vi "Multi_Run_Prog.vi"(0 "Command filename":path, 1 "Mode":T9(ring), 2 "Table":T6[](array[typedef]) {"Carrier_2 Q (l/min)" format="%#.2f"; "Row Duration (mins)" format="%#.1f"; "Row No" min=0; "Trace Gas Concentration (%)" min=0.0 format="%#_4f"; "Carrier_1 Q (l/min)" format="%#.2f"; "Tunnel Speed" format="%#.2f"; "Start X" format="%#.2f"; "Start Y" format="%#.2f"; "Start Z" format="%#.2f"; "End X" format="%#.2f"; "End Y" format="%#.2f"; "End Z" format="%#.2f"; "Averaging time (min)" min=0.0 format="%#.2f"}, 3 "Work in Tunnel Coordinates?":T1, 4 "Jump Bad Positions":bool) -> ()   [LabVIEW 2015]
uses:
  Anemometry Sub Vis/Gen Trav/Traverse_cluster.ctl
  Anemometry Sub Vis/Gen Trav/Spacing.ctl
  Anemometry Sub Vis/Controls/Multi_run_mode.ctl
  Anemometry Sub Vis/Gen Trav/Route mapping/Route_Display_Mode.ctl
  Anemometry Sub Vis/Controls/User_Specific_mode.ctl
  Anemometry Sub Vis/Controls/Multi_Run_Case.ctl
  Anemometry Sub Vis/Gen Trav/Multi_Run_Status.ctl
  Anemometry Sub Vis/Controls/Tunnel_Coordinates.ctl
  Anemometry Sub Vis/Controls/Post_Process.ctl
  ADAM Client/Sub VIs/ADAM Controls/Traverse_Level_State.ctl
  ADAM Client/Sub VIs/ADAM Controls/Tunnel_speed_mode.ctl
  Anemometry Sub Vis/Controls/Overhead.ctl
  ADAM Client/Sub VIs/ADAM Controls/Remember_value_mode.ctl
  Anemometry Sub Vis/Gen Trav/Trav_mode.ctl
  Anemometry Sub Vis/Controls/Home.ctl
  ADAM Client/Sub VIs/ADAM Controls/Client_Source_Status.ctl
  ADAM Client/Sub VIs/ADAM Controls/Update_scan_value.ctl
  Anemometry Sub Vis/File/Setup_Filetype.ctl
  Anemometry Sub Vis/Globals/Meas_global.vi
  Anemometry Sub Vis/Globals/Trav_pos_global.vi
  Anemometry Sub Vis/Globals/Preference_global.vi
  Anemometry Sub Vis/Gen Trav/Route mapping/Route_mapping_global.vi
  ADAM Serial/Instrument drivers/Traverses/~subVIs/DriveConfigGlobal.vi
  Anemometry Sub Vis/Globals/Extra_Commands_Global.vi
panel:
  in  "Sort Single\nMeasurements":bool
  out "Last Row Run":i32
  in  "Stop after Repeats":bool
  out "Current Overhead Factor":dbl format="%.3f"
  out "Estimated Completion time":string
  out "Max Tunnel Speed":dbl format="%.2f"
  out "Pause message":string
  in  "Pause":bool
  out "Non Starter":bool
  out "No of Rows":i32
  out "Status":T2
  in  "Synchronization Start No":i32=1 min=1 max=100
  out "Multi Run Case":T3
  out "Simulate/Run":T4
  in  "Display Mode":T5=enum."Display View on Crash"
  in  "stop":bool
  out "Currently on Row":i32
  # "X           Y            Z"
  # "Start"
  # "End"
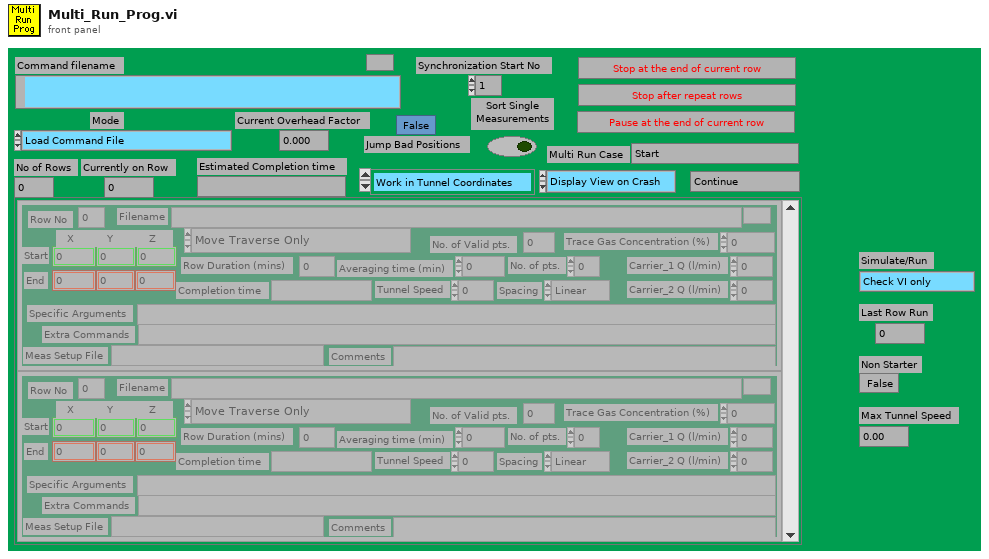
[diagram p1: front panel]
types:
  T1 = typedef "Tunnel_Coordinates.ctl" = enum16{"Work in Tunnel Coordinates", "Work in Model Coordinates"}
  T2 = typedef "Multi_Run_Status.ctl" = enum16{"Continue", "Jump to Next Point", "Jump to Next Row", "Jump To Fall Back", "Terminate Run"}
  T3 = typedef "Multi_Run_Case.ctl" = enum16{"Start", "Load Setup From File", "Has file been edited in Excel?", "Check Max Tunnel Speed", "Pre Check Row", "Check Rows", "Remove blank end rows", "Do results files already exist?", "FFID Bkgnd Measurements?", "First Save Setup file", "Setup Route checking", "Initialise Measurement Prog", "Input Current Position", "Experimental setup control", "Check source flowrates", "Setup for running mode", "Skip Blank Rows", "Which row to execute next", "Evaluate IF Statement", "Perform Measurement Setup", "Set Measurement Conditions", "Execute Row", "Calculate Row TIme", "Update time estimate", "Pause Multi Run Program", "Do Another Row?", "Find Next Fall Back Row", "Shut down source etc", "Email results to users", "Save run efficiency", "Remove Skipped Commands", "Show jumped positions", "Save Setup to File", "End"}
  T4 = typedef "User_Specific_mode.ctl" = enum16{"Check VI only", "Run VI"}
  T5 = typedef "Route_Display_Mode.ctl" = enum16{"Display View Always", "Display View on Crash"}
  T6 = typedef "Traverse_cluster.ctl" = cluster{"Start X":sgl, "Start Y":sgl, "Start Z":sgl, "End X":sgl, "End Y":sgl, "End Z":sgl, "No. of pts.":i32, "Spacing":T7, "Filename":path, "Tunnel Speed":dbl, "Averaging time (min)":dbl, "Extra Commands":string, "Carrier_1 Q (l/min)":dbl, "Carrier_2 Q (l/min)":dbl, "Trace Gas Concentration (%)":dbl, "Specific Arguments":string, "Comments":string, "Row No":i32, "Row Type Selector":T8, "Completion time":string, "Row Duration (mins)":dbl, "No. of Valid pts.":i32, "Meas Setup File":string}
  T7 = typedef "Spacing.ctl" = enum16{"Linear", "Log", "Gauss", "Specified", "N/A"}
  T8 = typedef "Multi_run_mode.ctl" = enum16{"Move Traverse Only", "Set Tunnel Speed Only", "Set Source Only", "Set Measurement Conditions", "Single Measurement", "Vertical Profile", "Lateral Profile", "Longitudinal Profile", "Explore Volume", "Multi-Axis Profile", "Auto Calibrate", "Meas Fast FID Bkgnd", "Check Beam Power", "Scanning Valve Measurement", "Run VI Named:", "Set ADAM Ch", "Wait (minutes)", "Send Message", "Synchronize With:", "Fall Back to this Row", "Turn Off Row Repeating", "Blank Row", "Traverse 3D Volume"}
  T9 = enum16{"Load Command File", "Save Command File", "Check Multi Run Prog", "Check Multi Run Prog With Live Moves", "Run Multi Run Prog"}
  T10 = typedef "Post_Process.ctl" = enum16{"Take New Data", "Post Process Raw Data File"}
  T11 = typedef "Traverse_Level_State.ctl" = enum16{"Running", "Complete"}
  T12 = enum32{"existing file", "new file", "new or existing file", "existing dir", "new dir", "new or existing dir", "existing file (use LLBs)", "new file (use LLBs)", "new or existing file (use LLBs)", "new or existing file or directory (use LLBs)"}
  T13 = typedef "Tunnel_speed_mode.ctl" = enum16{"Set Speed", "Set Speed then wait", "Is tunnel speed allowable?"}
  T14 = enum16{"All Channel Names", "Valid Channel Names"}
  T15 = typedef "Overhead.ctl" = enum16{"Update total times", "Read Current Overhead", "Re Scale totals to 3 hrs", "Initialise totals to 3hr"}
  T16 = typedef "Remember_value_mode.ctl" = enum16{"Read only", "Read and Write"}
  T17 = typedef "Home.ctl" = enum16{"Don't Home", "Home  +X", "Home  -X", "Home  +Y", "Home  -Y", "Home  +Z", "Home  -Z"}
  T18 = typedef "Trav_mode.ctl" = enum16{"Move traverse", "Read traverse position", "Teach Position"}
  T19 = typedef "Client_Source_Status.ctl" = enum16{"Not Using", "Using", "Must Have"}
  T20 = typedef "Update_scan_value.ctl" = cluster{"Channel Name":string, "New Value":dbl}
  T21 = typedef "Setup_Filetype.ctl" = enum16{"Measurement Setups", "Calibration Setups", "General", "Results File Plotter Setups", "Speed Calib Tweaks"}
  T22 = typedef "AxisConfigCluster.ctl" = cluster{"Channel Properties":T23, "Static Drive Configuration":T24}
  T23 = typedef "DriveProperties.ctl" = cluster{"Channel Name":string, "Vel. Default":sgl, "Acc. Default":sgl, "Vel. Max":sgl, "Vel. Min":sgl, "Acc. Max":sgl, "Acc. Min":sgl, "Pulses/unit":sgl, "Address":u8, "Pulse Offset":i32, "Pos Tolerance":sgl, "Pulses/rev":sgl, "Backlash/Eng units":sgl, "Current Pos":sgl, "Ch Status":enum16{"Active", "Offline", "Simulate"}, "Port Name":string, "Axis Transform mode":string, "Metadata Ch Name":string, "Type":string}
  T24 = typedef "DriveStaticConfig.ctl" = cluster{"Correction Gain % (CG)":u16, "Dead Band (DB)":i32, "Dead Band Window (DW)":i32, "Encoder Resolution (ER)":i32, "Step Mode  (FSB)":u16, "Position Maintenance (FSC)":u16, "Stop on Stall (FSD)":u16, "Activate OP1 on stall (FSE)":u16, "Stop on Trigger 3 (FSF)":u16, "OP2 in Deadband (FSG)":u16, "Stall Detect (FSH)":u16, "Limit Disable (LD)":u16, "Motor Resolution (MR)":enum16{"200", "400", "1000", "2000", "4000", "5000", "10000", "12800", "18000", "20000", "21600", "25000", "25400", "25600", "36000", "50000", "278528", "425984", "507904", "614400", "655360", "819200", "1024000"}, "Limit Switch Sense (OSA)":u16, "Home Position (OSB)":u16, "Home Switch Sense (OSC)":u16, "Encoder Z for Home (OSD)":u16, "Reference edge of Home (OSH)":u16, "RS232 Echo Control (SSA)":u16, "Buffer at Limit (SSG)":u16, "Buffer at Stop (SSH)":u16, "Indexer Mode  (FSA)":u16, "Type":string, "ConfigString":string, "De Power Motor":enum16{"TRUE", "FALSE"}}
  T25 = typedef "Status_Cluster.ctl" = cluster{"Status":T2, "Error Type":string, "Error Description":string}
  T26 = typedef "Server_Comms.ctl" = enum16{"Server Link Healthy", "Do Not Link To Server"}
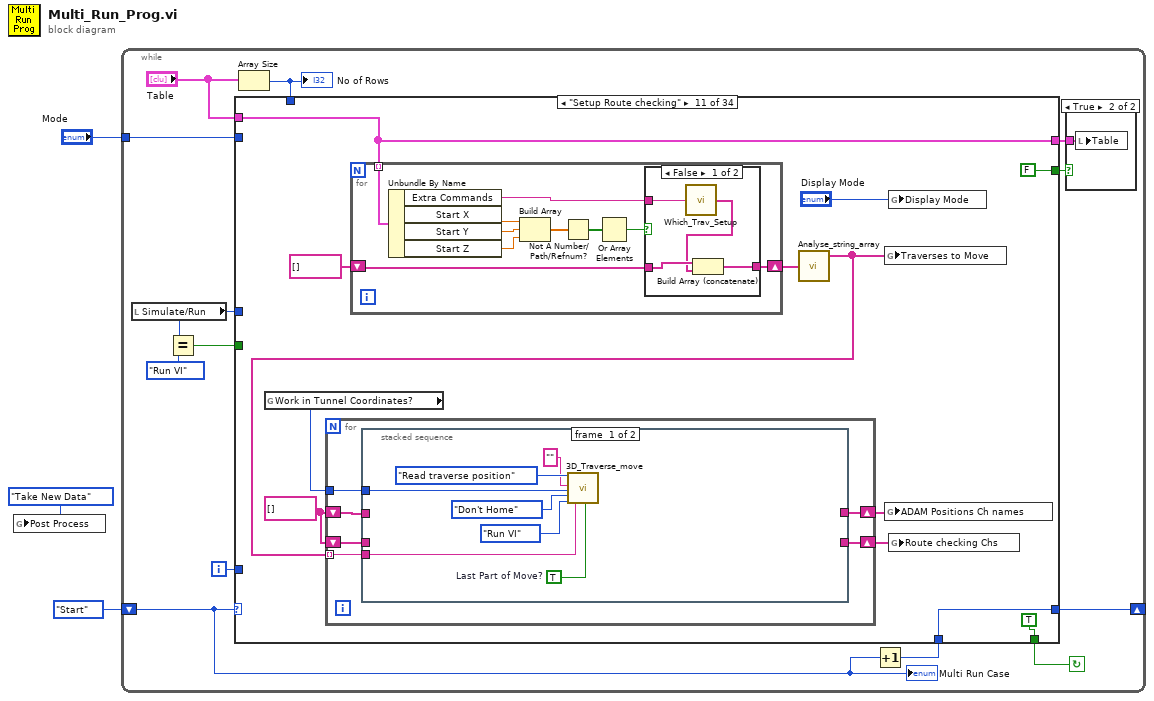
[diagram p0: block diagram]
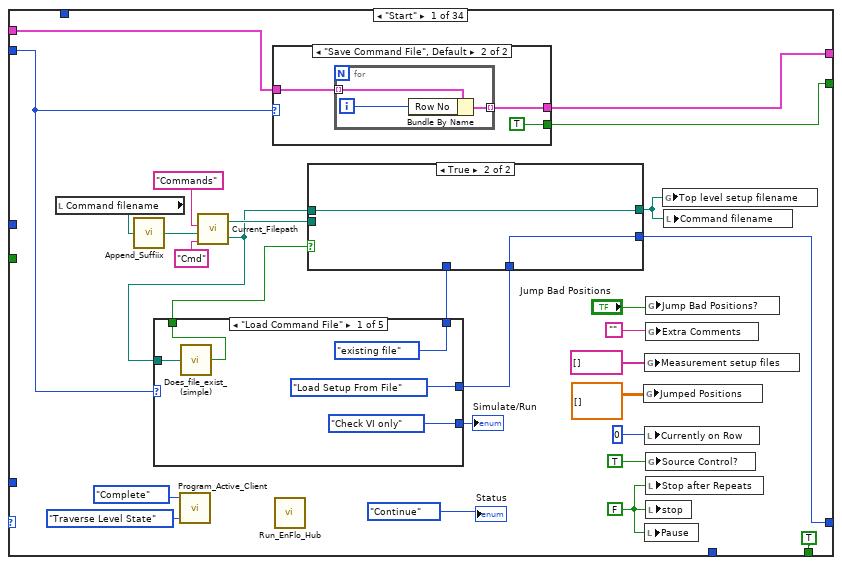
[diagram p3: hidden frame]
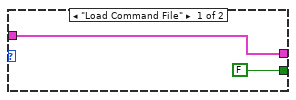
[diagram p4: hidden frame]
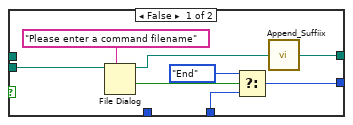
[diagram p5: hidden frame]
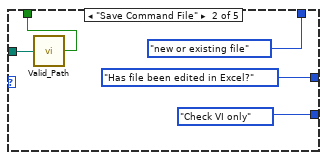
[diagram p6: hidden frame]
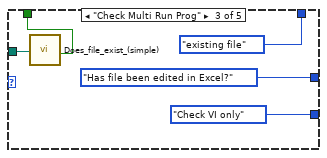
[diagram p7: hidden frame]
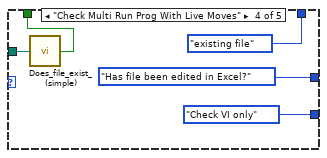
[diagram p8: hidden frame]
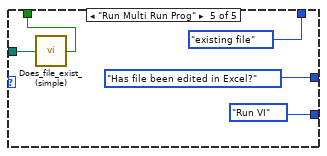
[diagram p9: hidden frame]
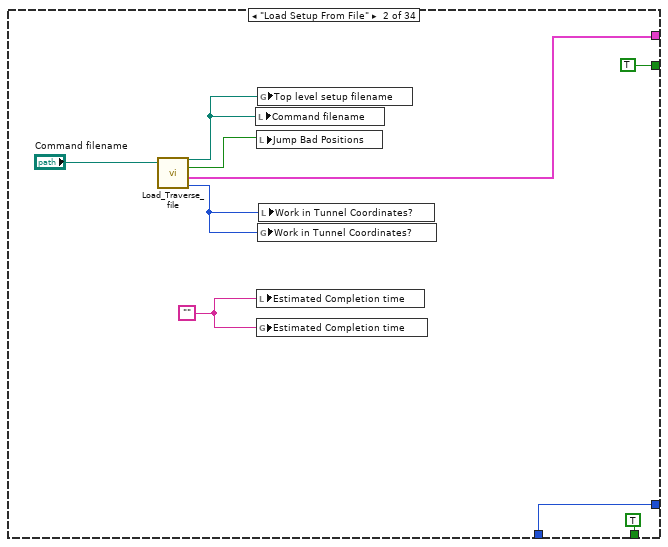
[diagram p10: hidden frame]
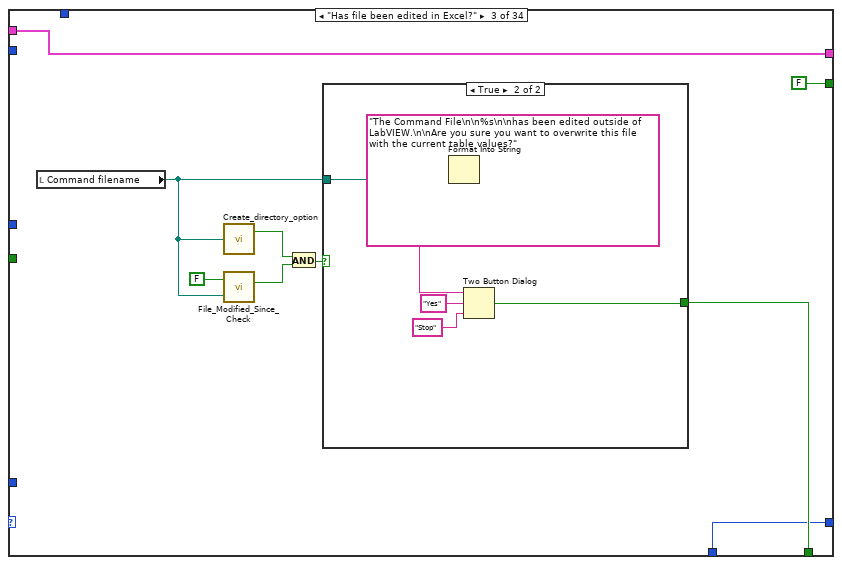
[diagram p11: hidden frame]
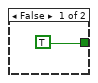
[diagram p12: hidden frame]
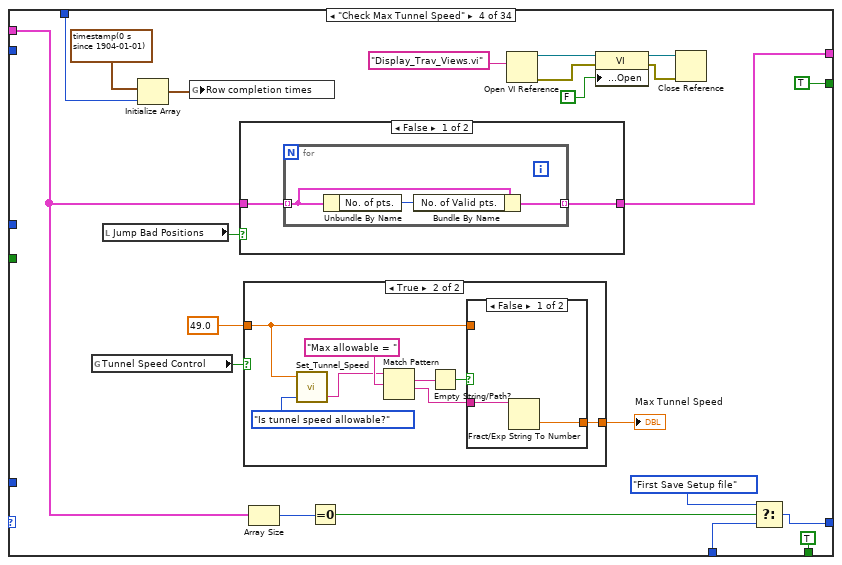
[diagram p13: hidden frame]
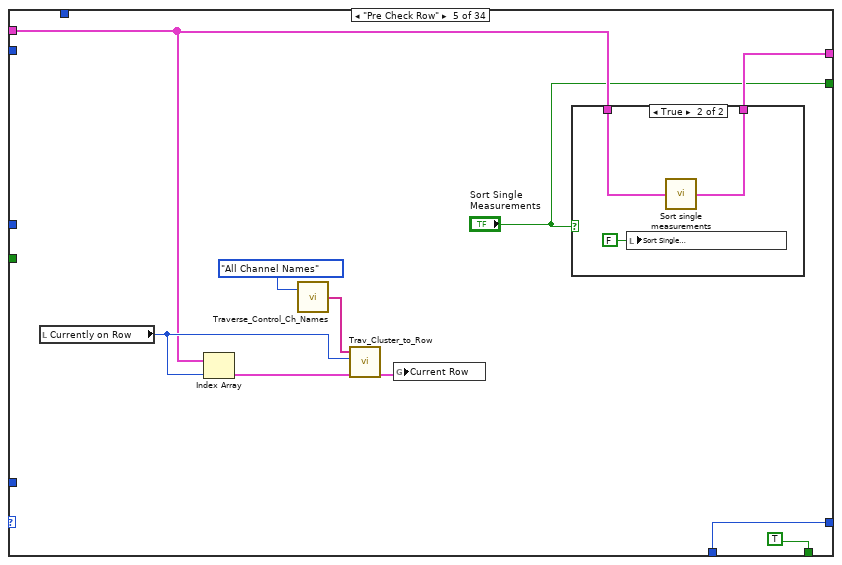
[diagram p17: hidden frame]
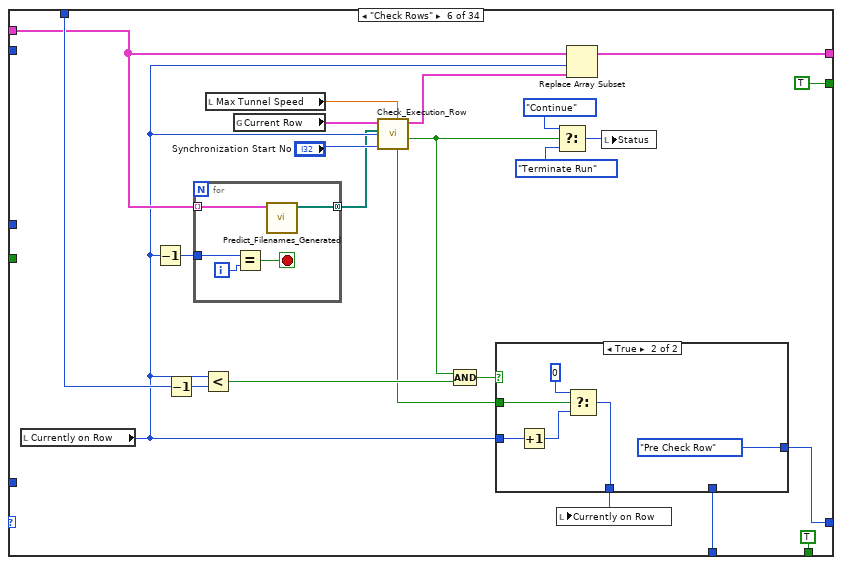
[diagram p19: hidden frame]
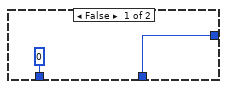
[diagram p20: hidden frame]
diagram:
  n1 = global write "Meas_global.vi" "Post Process"(Post_Process."Take New Data" ("Post Process")) -> ()
  n2 = while {
    shift-left: Multi_Run_Case."Start" ("Multi Run Case") -> [w12]
    shift-right: [w9] -> _
    tunnel: "Mode" -> [w15]
    i -> [w13]
    stop <- w16 continue-if-true
    n3 = local read "Simulate/Run"() -> (w5:T4)
    n4 = Equal?(x=w5, y=User_Specific_mode."Run VI" ("Simulate/Run")) -> (x = y?=w4:bool)
    n5 = Array Size(array="Table") -> (size(s)=w8:i32)
    "No of Rows" <- w8
    n6 = Increment(x=w12) -> (x+1=w14:T3)
    n7 = case shown="\"Setup Route checking\"" w12 {
      tunnel: [TRUE TRUE w100 TRUE TRUE TRUE TRUE TRUE TRUE TRUE TRUE ("Continue?") TRUE ("Continue?") TRUE TRUE TRUE w545 TRUE ("Continue?") TRUE ("Continue?") TRUE TRUE ("Continue?") TRUE TRUE TRUE TRUE TRUE TRUE TRUE TRUE TRUE TRUE TRUE TRUE TRUE FALSE] -> w16
      tunnel: w15 -> [w30 _ _ _ _ _ _ _ _ w426 _ _ _ _ _ _ _ _ _ _ _ _ _ _ _ _ _ _ _ _ _ _ w1268 _]
      tunnel: "Table" -> [w42 _ w97 w127 w155 w170 w204 w235 w393 w428 w451 w507 w519 w526 w534 w548 w610 w654 w758 w809 w821 w911 w945 w977 w1020 w1064 w1109 w1138 w1163 w1210 w1215 w1224 w1287 w1350]
      tunnel: w5 -> [_ _ _ _ _ _ _ w234 _ _ _ _ _ _ w533 w547 _ w652 _ w806 w818 w910 _ w974 _ w1070 _ _ _ _ _ _ w1278 _]
      tunnel: w14 -> [_ w93 w99 w125 w161 w176 w215 w238 w390 w425 w454 w505 w520 w525 w538 w550 w612 w650 w763 w810 w828 w908 w938 w979 w1023 _ _ w1124 w1165 w1212 w1218 w1232 w1285 w1349]
      tunnel: w13 -> [_ _ _ _ _ _ _ _ _ _ _ _ _ _ _ _ _ _ _ _ _ _ _ _ w1021 _ _ _ _ _ _ _ _ _]
      tunnel: [w40 w93 w99 w124 w161 w175 w215 w238 w390 w421 w454 w504 w520 w525 w536 w550 w612 w651 w762 w810 w829 w908 w938 w979 w1024 w1059 w1107 w1133 w1165 w1212 w1218 w1232 w1285 w1349] -> w9
      tunnel: [w29 TRUE FALSE ("Rows Added ?") TRUE ("Rows Added ?") "Sort Single\nMeasurements" TRUE TRUE FALSE FALSE TRUE FALSE FALSE FALSE FALSE FALSE TRUE FALSE ("Rows Added ?") FALSE ("Rows Added ?") FALSE FALSE ("Rows Added ?") FALSE FALSE FALSE TRUE ("Rows Added ?") FALSE FALSE FALSE FALSE FALSE FALSE TRUE TRUE TRUE FALSE] -> w10
      tunnel: w8 -> [_ _ _ w119 _ w180 w206 _ _ _ _ _ _ _ _ _ w613 w653 _ _ _ _ _ w973 _ w1062 w1100 _ _ _ _ _ w1259 _]
      tunnel: [w41 w94 w97 w129 w154 w183 w210 w235 w393 w429 w451 w507 w519 w526 w534 w546 w610 w655 w758 w809 w821 w911 w945 w976 w1020 w1064 w1109 w1138 w1163 w1210 w1214 w1224 w1286 w1350] -> w7
      tunnel: w4 -> [_ _ _ _ _ _ _ _ _ _ _ _ _ w523 w532 _ _ _ w752 _ _ _ w937 _ _ _ _ _ _ _ _ _ _ _]
      frame "Start" {
        w27 = FALSE ("Measurment setup Found?")
        n8 = local read "Command filename"() -> (w32:path)
        n9 = call "Append_Suffiix.vi"("Results file"=w32) -> ("appended path"=w22:path)
        n10 = call "Program_Active_Client.vi"("Mode"=enum16{"Program Active", "Traverse Level State"}."Traverse Level State", "Traverse level State"=Traverse_Level_State."Complete") -> ()  [unwired: 1 in, 3 out]
        n11 = call "Current_Filepath.vi"("Short_Name"="Cmd" ("Data Type"), "Filename in"=w22, "Data Type"="Commands") -> ("Filename Out"=w19:path, "Directory"=w21:path)  [unwired: 1 in]
        n12 = case shown="\"Load Command File\"" w30 {
          tunnel: [User_Specific_mode."Check VI only" ("Simulate/Run") User_Specific_mode."Check VI only" ("Simulate/Run") User_Specific_mode."Check VI only" ("Simulate/Run") User_Specific_mode."Check VI only" ("Simulate/Run") User_Specific_mode."Run VI" ("Simulate/Run")] -> w43
          tunnel: [Multi_Run_Case."Load Setup From File" ("Multi Run Case") Multi_Run_Case."Has file been edited in Excel?" ("Multi Run Case") Multi_Run_Case."Has file been edited in Excel?" ("Multi Run Case") Multi_Run_Case."Has file been edited in Excel?" ("Multi Run Case") Multi_Run_Case."Has file been edited in Excel?" ("Multi Run Case")] -> w39
          tunnel: [T12."existing file" ("select mode (2)") T12."new or existing file" ("select mode (2)") T12."existing file" ("select mode (2)") T12."existing file" ("select mode (2)") T12."existing file" ("select mode (2)")] -> w28
          tunnel: w19 -> [w64 w69 w73 w79 w84]
          tunnel: [w63 w68 w74 w78 w83] -> w18
          frame "Load Command File" {
            n13 = call "Does_file_exist_(simple).vi"("Pathname"=w64) -> ("exists?"=w63:bool)
          }
          frame "Save Command File" {
            n14 = call "Valid_Path.vi"("Filename"=w69) -> ("Valid Path?"=w68:bool)
          }
          frame "Check Multi Run Prog" {
            n15 = call "Does_file_exist_(simple).vi"("Pathname"=w73) -> ("exists?"=w74:bool)
          }
          frame "Check Multi Run Prog With Live Moves" {
            n16 = call "Does_file_exist_(simple).vi"("Pathname"=w79) -> ("exists?"=w78:bool)
          }
          frame "Run Multi Run Prog" {
            n17 = call "Does_file_exist_(simple).vi"("Pathname"=w84) -> ("exists?"=w83:bool)
          }
        }
        "Simulate/Run" <- w43
        n18 = case shown="\"Save Command File\", Default" w30 {
          tunnel: w42 -> [w46 w49]
          tunnel: [w46 w48] -> w41
          tunnel: [FALSE TRUE] -> w29
          frame "Load Command File" {
          }
          frame "Save Command File", Default {
            n19 = for {
              tunnel: w49 -> [w52] mode=indexing
              tunnel: [w51] -> w48 mode=indexing
              i -> [w50]
              n20 = Bundle By Name(cluster=w52, "Row No"=w50) -> (w51:T6)
            }
          }
        }
        n21 = call "Run_EnFlo_Hub.vi"() -> ()  [unwired: 8 out]
        n22 = case shown="True" w18 {
          tunnel: [w58 w62] -> w40
          tunnel: w39 -> [w59 w62]
          tunnel: w19 -> [_ w61]
          tunnel: [w57 w61] -> w31
          tunnel: w28 -> [_ _]
          tunnel: w21 -> [w53 _]
          frame False {
            n23 = File Dialog(7:"Please enter a command filename" ("prompt"), 11:w53) -> (1:w55:bool, 3:w56:path)  [unwired: 1 in, 6 out]
            n24 = Select(t=Multi_Run_Case."End" ("Multi Run Case"), s=w55, f=w59) -> (s? t:f=w58:T3)
            n25 = call "Append_Suffiix.vi"("Results file"=w56) -> ("appended path"=w57:path)
          }
          frame True {
          }
        }
        n26 = global write "Trav_pos_global.vi" "Jumped Positions"(dbl[][] [] ("Jumped Positions")) -> ()
        n27 = global write "Trav_pos_global.vi" "Measurement setup files"(string[] [] ("Measurement setup files")) -> ()
        n28 = local write "Currently on Row"(0 ("Currently on Row")) -> ()
        n29 = local write "Pause"(w27) -> ()
        n30 = global write "Trav_pos_global.vi" "Jump Bad Positions?"("Jump Bad Positions") -> ()
        n31 = global write "Meas_global.vi" "Extra Comments"("") -> ()
        n32 = global write "Trav_pos_global.vi" "Source Control?"(TRUE ("Source Control?")) -> ()
        n33 = local write "Stop after Repeats"(w27) -> ()
        n34 = local write "stop"(w27) -> ()
        n35 = global write "Trav_pos_global.vi" "Top level setup filename"(w31) -> ()
        n36 = local write "Command filename"(w31) -> ()
        "Status" <- Multi_Run_Status."Continue" ("Status")
      }
      frame "Load Setup From File" {
        w89 = ""
        n37 = call "Load_Traverse_file.vi"("Setup filename"="Command filename") -> ("Setup filename Out"=w91:path, "Jump Bad Positions"=w88:bool, "Table"=w94:T6[], "Work in Tunnel Coordinates?"=w90:T1)  [unwired: 2 out]
        n38 = local write "Command filename"(w91) -> ()
        n39 = local write "Jump Bad Positions"(w88) -> ()
        n40 = local write "Estimated Completion time"(w89) -> ()
        n41 = global write "Trav_pos_global.vi" "Estimated Completion time"(w89) -> ()
        n42 = global write "Trav_pos_global.vi" "Top level setup filename"(w91) -> ()
        n43 = global write "Trav_pos_global.vi" "Work in Tunnel Coordinates?"(w90) -> ()
        n44 = local write "Work in Tunnel Coordinates?"(w90) -> ()
      }
      frame "Has file been edited in Excel?" {
        n45 = local read "Command filename"() -> (w101:path)
        n46 = call "Create_directory_option.vi"("Filename"=w101) -> ("Path is to existing File"=w104:bool)  [unwired: 1 out]
        n47 = call "File_Modified_Since_Check.vi"("Pathname"=w101, "Just Modified?"=FALSE) -> ("Modified?"=w103:bool)
        n48 = And(x=w104, y=w103) -> (x .and. y?=w105:bool)
        n49 = case shown="True" w105 {
          tunnel: w101 -> [_ w112]
          tunnel: [TRUE ("T button?") w107] -> w100
          frame False {
          }
          frame True {
            n50 = Format Into String(format string="The Command File\n\n%s\n\nhas been edited outside of LabVIEW.\n\nAre you sure you want to overwrite this file  with the current table values?" ("Format String"), w112) -> (resulting string=w110:string)  [unwired: 2 in, 1 out]
            n51 = Two Button Dialog(message=w110, 1:"Stop" ("F button name (\"Cancel\")"), 2:"Yes" ("T button name (\"OK\")")) -> (T button?=w107:bool)
          }
        }
      }
      frame "Check Max Tunnel Speed" {
        n52 = global read "Preference_global.vi" "Tunnel Speed Control"() -> (w130:bool)
        n53 = local read "Jump Bad Positions"() -> (w128:bool)
        n54 = Initialize Array(timestamp(0 s since 1904-01-01) ("seconds since 1Jan1904"), w119) -> (w120:timestamp[])
        n55 = global write "Trav_pos_global.vi" "Row completion times"(w120) -> ()
        n56 = case shown="False" w128 {
          tunnel: w127 -> [w136 w140]
          tunnel: [w135 w140] -> w129
          frame False {
            n57 = for {
              tunnel: w136 -> [w138] mode=indexing
              tunnel: [w137] -> w135 mode=indexing
              n58 = Unbundle By Name(w138) -> ("No. of pts."=w139:i32)
              n59 = Bundle By Name(cluster=w138, "No. of Valid pts."=w139) -> (w137:T6)
            }
          }
          frame True {
          }
        }
        n60 = case shown="True" w130 {
          tunnel: 49.0 ("Tunnel Velocity m/s") -> [w141 w142]
          tunnel: [w141 w144] -> w132
          frame False {
          }
          frame True {
            n61 = call "Set_Tunnel_Speed.vi"("Mode"=Tunnel_speed_mode."Is tunnel speed allowable?", "Tunnel Velocity m/s"=w142) -> ("Error String"=w147:string)  [unwired: 1 in, 2 out]
            n62 = Match Pattern(string=w147, regular expression="Max allowable = ") -> (match substring=w146:string, after substring=w143:string)  [unwired: 3 out]
            n63 = Empty String/Path?(string/path=w146) -> (empty?=w145:bool)
            n64 = case shown="False" w145 {
              tunnel: [w150 w152] -> w144
              tunnel: w142 -> [_ w152]
              tunnel: w143 -> [w151 _]
              frame False {
                n65 = Fract/Exp String To Number(string=w151) -> (number=w150:dbl)  [unwired: 4 out]
              }
              frame True {
              }
            }
          }
        }
        "Max Tunnel Speed" <- w132
        n66 = Array Size(array=w127) -> (size(s)=w126:i32)
        n67 = Equal To 0?(x=w126) -> (x = 0?=w123:bool)
        n68 = Open VI Reference(vi path="Display_Trav_Views.vi" ("VI path")) -> (vi reference=w118:refnum<vi>, error out=w117:errorcluster)  [unwired: 1 in, 4 out]
        n69 = property class="VI"(reference=w118, error in=w117, "Front Panel Window:Open"=FALSE) -> (reference out=w115:refnum<vi>, error out=w114:errorcluster)
        n70 = Close Reference(reference=w115, error in (no error)=w114) -> ()  [unwired: 1 out]
        n71 = Select(t=Multi_Run_Case."First Save Setup file" ("Multi Run Case"), s=w123, f=w125) -> (s? t:f=w124:T3)
      }
      frame "Pre Check Row" {
        n72 = local read "Currently on Row"() -> (w158:i32)
        n73 = Index Array(array=w155, index=w158) -> (element=w159:T6)
        n74 = call "Traverse_Control_Ch_Names.vi"("Mode"=T14."All Channel Names") -> ("Channel names"=w156:string[])  [unwired: 1 in]
        n75 = call "Trav_Cluster_to_Row.vi"("Traverse line in"=w159, "Row Number"=w158, "Channel names"=w156) -> ("Traverse line Out"=w160:T6)  [unwired: 4 out]
        n76 = global write "Trav_pos_global.vi" "Current Row"(w160) -> ()
        n77 = case shown="True" "Sort Single\nMeasurements" {
          tunnel: w155 -> [w163 w166]
          tunnel: [w163 w165] -> w154
          frame False {
          }
          frame True {
            n78 = local write "Sort Single\nMeasurements"(FALSE ("Sort Single\nMeasurements")) -> ()
            n79 = call "Sort single measurements.vi"("Table In"=w166) -> ("Table Out"=w165:T6[])
          }
        }
      }
      frame "Check Rows" {
        n80 = local read "Currently on Row"() -> (w169:i32)
        n81 = Decrement(x=w169) -> (x-1=w168:i32)
        n82 = Decrement(x=w180) -> (x-1=w173:i32)
        n83 = for {
          tunnel: w170 -> [w194] mode=indexing
          tunnel: w168 -> [w192]
          tunnel: [w190] -> w167 mode=concatenating
          i -> [w193]
          stop <- w191 stop-if-true
          n84 = Equal?(x=w192, y=w193) -> (x = y?=w191:bool)
          n85 = call "Predict_Filenames_Generated.vi"("Traverse line"=w194) -> ("Filename"=w190:path[])  [unwired: 10 in]
        }
        n86 = Less?(x=w169, y=w173) -> (x < y?=w179:bool)
        n87 = local read "Max Tunnel Speed"() -> (w182:dbl)
        n88 = global read "Trav_pos_global.vi" "Current Row"() -> (w171:T6)
        n89 = call "Check_Execution_Row.vi"("Execution Row"=w171, "Earlier Filenames"=w167, "Synchronization Start No"="Synchronization Start No", "Row Index"=w169, "Max Tunnel Speed"=w182) -> ("Edited Row"=w172:bool, "Execution Row Out"=w174:T6, "Continue?"=w181:bool)  [unwired: 3 out]
        n90 = Compound Arithmetic op=AND(w181, w179) -> (w178:bool)
        n91 = case shown="True" w178 {
          tunnel: [0 w198] -> w177
          tunnel: w169 -> [_ w202]
          tunnel: w176 -> [w196 _]
          tunnel: [w196 Multi_Run_Case."Pre Check Row" ("Multi Run Case")] -> w175
          tunnel: w172 -> [_ w200]
          frame False {
          }
          frame True {
            n92 = Increment(x=w202) -> (x+1=w199:i32)
            n93 = Select(t=0, s=w200, f=w199) -> (s? t:f=w198:i32)
          }
        }
        n94 = Select(t=Multi_Run_Status."Continue" ("Status"), s=w181, f=Multi_Run_Status."Terminate Run" ("Status")) -> (s? t:f=w187:T2)
        n95 = local write "Currently on Row"(w177) -> ()
        n96 = Replace Array Subset(array=w170, new element=w174, index=w169) -> (w183:T6[])
        n97 = local write "Status"(w187) -> ()
      }
      frame "Remove blank end rows" {
        n98 = local read "Jump Bad Positions"() -> (w203:bool)
        n99 = case shown="False" w203 {
          tunnel: w206 -> [w221 _]
          tunnel: w204 -> [w220 w224]
          tunnel: [w218 w224] -> w205
          frame False {
            n100 = call "Calc_Remaining_Time.vi"("Currently on Row"=-1 ("Start Index"), "Table In"=w220) -> ("Table Out"=w218:T6[])  [unwired: 1 out]
            n101 = Decrement(x=w221) -> (x-1=w223:i32)
            n102 = Index Array(array=w218, index=w223) -> (element=w222:T6)
            n103 = Unbundle By Name(w222) -> ("Completion time"=w217:string)
            n104 = global write "Trav_pos_global.vi" "Estimated Completion time"(w217) -> ()
            n105 = local write "Estimated Completion time"(w217) -> ()
          }
          frame True {
          }
        }
        n106 = Reverse 1D Array(array=w205) -> (reversed array=w214:T6[])
        n107 = while {
          tunnel: [w225] -> w212
          tunnel: w206 -> [w229]
          tunnel: w214 -> [w233] mode=indexing
          i -> [w225]
          stop <- w226 continue-if-true
          n108 = Unbundle By Name(w233) -> ("Row Type Selector"=w231:T8)
          n109 = Increment(x=w225) -> (x+1=w230:i32)
          n110 = Greater?(x=w229, y=w230) -> (0:w228:bool)
          n111 = Equal?(x=Multi_run_mode."Blank Row" ("Row Type Selector"), y=w231) -> (x = y?=w227:bool)
          n112 = And(x=w227, y=w228) -> (x .and. y?=w226:bool)
        }
        n113 = Subtract(x=w206, y=w212) -> (x-y=w211:i32)
        n114 = call "Overhead_Factor.vi"("Mode"=Overhead."Read Current Overhead") -> ("Current Overhead Factor"=w207:dbl)  [unwired: 3 in]
        n115 = local write "Current Overhead Factor"(w207) -> ()
        n116 = Array Subset(array=w205, index=0 ("Array Index"), length=w211) -> (w210:T6[])
      }
      frame "Do results files already exist?" {
        n117 = for {
          tunnel: w235 -> [w247] mode=indexing
          shift-right: [w243] -> _
          shift-left: path[] [] -> [w244]
          tunnel: w234 -> [w241]
          n118 = Unbundle By Name(w247) -> ("Specific Arguments"=w240:string, "Row Type Selector"=w246:T8, "Filename"=w245:path)
          n119 = while {
            shift-left: w244 -> [w255]
            shift-right: [w254] -> w243
            tunnel: w245 -> [w256]
            tunnel: w246 -> [w260]
            shift-left: 0 -> [w261]
            shift-right: [w257] -> _
            tunnel: w241 -> [w251]
            shift-right: [w250] -> _
            shift-left: _ -> [w249]
            tunnel: w240 -> [w248]
            stop <- w259 continue-if-true
            n120 = Increment(x=w261) -> (x+1=w258:i32)
            n121 = case shown="0, Default" w261 {
              tunnel: w260 -> [w270 _ _ _ _ _ _ _ _ _ _ _]
              tunnel: [w265 w292 w297 w304 w309 TRUE ("exists?") TRUE ("exists?") FALSE ("exists?") FALSE ("exists?") TRUE ("true") w366 w379] -> w259
              tunnel: w258 -> [w272 w295 w300 w303 w310 w315 w326 w337 w348 w352 w364 _]
              tunnel: [w272 w295 w300 w303 w310 w313 w325 w337 w348 w353 w364 w378] -> w257
              tunnel: [w271 w294 w299 w302 w307 w323 w334 w339 w341 w350 w368 w384] -> w254
              tunnel: w255 -> [w271 w294 w299 w302 w308 w323 w334 w339 w341 w350 w368 w384]
              tunnel: w256 -> [w264 _ _ _ _ _ _ _ _ _ _ _]
              tunnel: 7 -> [_ _ _ _ _ _ _ _ _ w351 _ w378]
              tunnel: 9 -> [_ _ _ _ _ w314 _ _ _ _ _ _]
              tunnel: w251 -> [_ _ _ _ _ _ _ _ _ _ w367 _]
              tunnel: [w263 w291 w296 w301 w306 w311 w324 w335 w340 w349 w365 w377] -> w250
              tunnel: w249 -> [_ w291 w296 w301 w306 w311 w324 w335 w340 w349 w365 w377]
              tunnel: w248 -> [w262 _ _ _ _ _ _ _ _ _ _ _]
              frame 0, Default {
                n122 = case shown="\"Run VI Named:\"" w270 {
                  tunnel: [TRUE w283 FALSE FALSE] -> w267
                  tunnel: w264 -> [w273 w282 w287 w289]
                  tunnel: w262 -> [_ w280 _ _]
                  tunnel: [w273 w282 w287 w289] -> w263
                  frame "Move Traverse Only", Default {
                  }
                  frame "Run VI Named:" {
                    n123 = Match Pattern(string=w280, regular expression=";") -> (before substring=w279:string)  [unwired: 4 out]
                    n124 = call <vilib>:"Trim Whitespace.vi"("string"=w279) -> ("trimmed string"=w277:string)  [unwired: 1 in]
                    n125 = Equal?(x=w277, y="Pressure_Tapped_Cube.vi") -> (x = y?=w284:bool)
                    n126 = Equal?(x=w277, y="Take_Data_on_the_Move.vi") -> (x = y?=w278:bool)
                    n127 = Equal?(x=w277, y="Capture_Flow_Vis.vi") -> (x = y?=w275:bool)
                    n128 = Compound Arithmetic op=OR(w284, w278, w275) -> (w283:bool)
                  }
                  frame "Auto Calibrate" {
                  }
                  frame "Send Message" {
                  }
                }
                n129 = local read "Status"() -> (w268:T2)
                n130 = Not Equal?(x=Multi_Run_Status."Terminate Run" ("Status"), y=w268) -> (x != y?=w266:bool)
                n131 = And(x=w267, y=w266) -> (x .and. y?=w265:bool)
              }
              frame 1 {
                n132 = Not Equal?(x=path "", y=w291) -> (x != y?=w292:bool)
              }
              frame 2 {
                n133 = Not Equal?(x=w296, y=path "") -> (x != y?=w297:bool)
              }
              frame 3 {
                n134 = Search 1D Array(1D array=w302, element=w301) -> (index of element=w305:i32)  [unwired: 1 out]
                n135 = Less Than 0?(x=w305) -> (x < 0?=w304:bool)
              }
              frame 4 {
                n136 = Build Array (concatenate)(w308, w306) -> (w307:path[])
                n137 = call "Does_file_exist_(simple).vi"("Pathname"=w306) -> ("exists?"=w309:bool)
              }
              frame 5 {
                n138 = Path To String(path=w311) -> (string=w322:string)
                n139 = global read "Meas_global.vi" "Start Time of experiment"() -> (w317:dbl)
                n140 = Concatenate Strings(w322, "Append" ("Substring")) -> (w320:string)
                n141 = call "Remember_value.vi"("Mode"=Remember_value_mode."Read only", "Ch name"=w320) -> ("Output Value"=w318:dbl)  [unwired: 1 in]
                n142 = Not Equal?(x=w317, y=w318) -> (x != y?=w316:bool)
                n143 = Select(t=w315, s=w316, f=w314) -> (s? t:f=w313:i32)
              }
              frame 6 {
                n144 = Increment(x=w326) -> (x+1=w327:i32)
                n145 = Format Into String(format string="The results filename \"%s\" already exists.\nDo you wish to append to this file during the run?" ("Format String"), w324) -> (resulting string=w331:string)  [unwired: 2 in, 1 out]
                n146 = Two Button Dialog(message=w331, 1:"Abort Run" ("F button name (\"Cancel\")"), 2:"Append" ("T button name (\"OK\")")) -> (T button?=w328:bool)
                n147 = Select(t=w327, s=w328, f=w326) -> (s? t:f=w325:i32)
              }
              frame 7 {
                n148 = local write "Status"(Multi_Run_Status."Terminate Run" ("Status")) -> ()
              }
              frame 8 {
                n149 = Path To String(path=w340) -> (string=w347:string)
                n150 = Concatenate Strings(w347, "Append" ("Substring")) -> (w345:string)
                n151 = global read "Meas_global.vi" "Start Time of experiment"() -> (w342:dbl)
                n152 = call "Remember_value.vi"("Mode"=Remember_value_mode."Read and Write", "Input Value"=w342, "Ch name"=w345) -> ()  [unwired: 1 out]
              }
              frame 9 {
                n153 = call "Read_File_Simple.vi"("Filename"=w349) -> ("string"=w356:string)  [unwired: 2 in, 7 out]
                n154 = call "Is_it_a_Results_File.vi"("character string"=w356) -> ("Results File?"=w355:bool)  [unwired: 2 out]
                n155 = case shown="False" w355 {
                  tunnel: w349 -> [w359 _]
                  tunnel: [w357 w363] -> w353
                  tunnel: w352 -> [_ w363]
                  tunnel: w351 -> [w357 _]
                  frame False {
                    n156 = Path To String(path=w359) -> (string=w361:string)
                    n157 = Format Into String(format string="The File %s is not in the correct Results file format.\nCheck that it is tab delimited rather than excel format, or choose another file." ("Format String"), w361) -> (resulting string=w358:string)  [unwired: 2 in, 1 out]
                    n158 = One Button Dialog(message=w358, button name ("OK")="Stop") -> ()  [unwired: 1 out]
                  }
                  frame True {
                  }
                }
              }
              frame 10 {
                n159 = case shown="\"Run VI\"" w367 {
                  tunnel: w365 -> [_ w376]
                  tunnel: [FALSE ("exists?") w370] -> w366
                  frame "Check VI only", Default {
                  }
                  frame "Run VI" {
                    n160 = call "Open_File_for_write.vi"("append to file? (new file:F)"=TRUE, "file path"=w376) -> ("error out"=w374:errorcluster, "refnum"=w375:refnum<file>)  [unwired: 1 in, 7 out]
                    n161 = Unbundle By Name(w374) -> ("code"=w373:i32)
                    n162 = Close File(refnum=w375, error in=w374) -> ()  [unwired: 2 out]
                    n163 = Equal?(x=10 ("code"), y=w373) -> (x = y?=w370:bool)
                  }
                }
              }
              frame 11 {
                n164 = Path To String(path=w377) -> (string=w382:string)
                n165 = Format Into String(format string="The File %s is already open in another application." ("Format String"), w382) -> (resulting string=w381:string)  [unwired: 2 in, 1 out]
                n166 = One Button Dialog(message=w381, button name ("OK")="Stop") -> (true=w379:bool)
              }
            }
          }
        }
      }
      frame "FFID Bkgnd Measurements?" {
        n167 = for {
          tunnel: w393 -> [w406] mode=indexing
          tunnel: [w404] -> w392 mode=indexing
          tunnel: [w403] -> w391 mode=indexing
          tunnel: [w401] -> w386 mode=indexing
          n168 = Unbundle By Name(w406) -> ("Specific Arguments"=w402:string, "Carrier_1 Q (l/min)"=w399:dbl, "Carrier_2 Q (l/min)"=w398:dbl, "Row Type Selector"=w400:T8)
          n169 = Add(x=w399, y=w398) -> (x+y=w397:dbl)
          n170 = case shown="\"Auto Calibrate\"" w400 {
            tunnel: w397 -> [w409 _]
            tunnel: [FALSE w410] -> w403
            tunnel: w402 -> [_ w411]
            tunnel: [w408 w410] -> w401
            frame Default {
              n171 = Greater Than 0?(x=w409) -> (x > 0?=w408:bool)
            }
            frame "Auto Calibrate" {
              n172 = call "Get_array_values_fr_String.vi"("String Value"=w411) -> ("String array"=w414:string[])  [unwired: 1 out]
              n173 = Index Array(array=w414, index=0 ("Index")) -> (element=w413:string)
              n174 = Equal?(x=w413, y="Concentration") -> (x = y?=w410:bool)
            }
          }
          n175 = Equal?(x=Multi_run_mode."Meas Fast FID Bkgnd" ("Row Type Selector"), y=w400) -> (x = y?=w404:bool)
        }
        n176 = Or Array Elements(Boolean array=w392) -> (logical OR=w388:bool)
        n177 = Or Array Elements(Boolean array=w386) -> (logical OR=w385:bool)
        n178 = Or Array Elements(Boolean array=w391) -> (logical OR=w387:bool)
        n179 = global write "Trav_pos_global.vi" "Source Control?"(w385) -> ()
        n180 = Compound Arithmetic op=AND(w387, invert w388) -> (w389:bool)
        n181 = case shown="True" w389 {
          frame False {
          }
          frame True {
            n182 = One Button Dialog(message="This run automatically calibrates the Fast FID but does not have a Meas Fast FID Bkgnd row" ("format string")) -> ()  [unwired: 2 out]
          }
        }
      }
      frame "First Save Setup file" {
        w416 = -1 ("Currently on Row")
        n183 = global write "Trav_pos_global.vi" "Work in Tunnel Coordinates?"("Work in Tunnel Coordinates?") -> ()
        n184 = case shown="\"Save Command File\"" w426 {
          tunnel: [w433 w435 w437 Multi_Run_Case."End" ("Multi Run Case") Multi_Run_Case."End" ("Multi Run Case")] -> w420
          tunnel: w425 -> [w433 w435 w437 _ _]
          tunnel: [w434 w436 w438 w439 w441] -> w419
          frame "Run Multi Run Prog" {
            w434 = FALSE  # Live Traverse Preview?
          }
          frame "Check Multi Run Prog With Live Moves" {
            w436 = TRUE  # Live Traverse Preview?
          }
          frame "Check Multi Run Prog" {
            w438 = FALSE  # Live Traverse Preview?
          }
          frame "Load Command File" {
            w439 = FALSE  # Live Traverse Preview?
          }
          frame "Save Command File" {
            w441 = FALSE  # Live Traverse Preview?
          }
        }
        n185 = local read "Command filename"() -> (w427:path)
        n186 = local read "Jump Bad Positions"() -> (w417:bool)
        n187 = call "Save_Trav_setup.vi"("Work in Tunnel Coordinates?"="Work in Tunnel Coordinates?", "Trav Table"=w428, "Jump Bad Positions"=w417, "Setup filename"=w427) -> ("Trav Table Out"=w429:T6[])  [unwired: 1 out]
        n188 = local read "Status"() -> (w422:T2)
        n189 = global write "Meas_global.vi" "Extra Comments"("") -> ()
        n190 = local write "Currently on Row"(w416) -> ()
        n191 = local write "Last Row Run"(w416) -> ()
        n192 = case shown="\"Continue\"" w422 {
          tunnel: [w431 Multi_Run_Case."End" ("Multi Run Case")] -> w421
          tunnel: w420 -> [w431 _]
          frame "Continue" {
          }
          frame "Jump to Next Point", Default {
          }
        }
        n193 = global write "Trav_pos_global.vi" "Live Traverse Preview?"(w419) -> ()
      }
      frame "Setup Route checking" {
        w447 = string[] []
        n194 = global read "Trav_pos_global.vi" "Work in Tunnel Coordinates?"() -> (w448:T1)
        n195 = for {
          tunnel: w451 -> [w493] mode=indexing
          shift-right: [w484] -> w449
          shift-left: string[] [] -> [w485]
          n196 = Unbundle By Name(w493) -> ("Extra Commands"=w486:string, "Start X"=w490:sgl, "Start Y"=w489:sgl, "Start Z"=w488:sgl)
          n197 = Build Array(w490, w489, w488) -> (w491:sgl[])
          n198 = Not A Number/Path/Refnum?(number/path/refnum=w491) -> (NaN/Path/Refnum?=w492:bool[])
          n199 = Or Array Elements(Boolean array=w492) -> (logical OR=w487:bool)
          n200 = case shown="False" w487 {
            tunnel: w486 -> [w497 _]
            tunnel: w485 -> [w496 w498]
            tunnel: [w495 w498] -> w484
            frame False {
              n201 = call "Which_Trav_Setup.vi"("Extra Command String"=w497) -> ("Traverse Setups"=w494:string[])
              n202 = Build Array (concatenate)(w496, w494) -> (w495:string[])
            }
            frame True {
            }
          }
        }
        n203 = call "Analyse_string_array.vi"("String array"=w449) -> ("Unique strings"=w444:string[])  [unwired: 2 out]
        n204 = for {
          tunnel: w444 -> [w460] mode=indexing
          tunnel: w448 -> [w459]
          shift-right: [w458] -> w445
          shift-left: w447 -> [w457]
          shift-right: [w455] -> w446
          shift-left: w447 -> [w456]
          n205 = stacked-sequence {
            tunnel: w460 -> [w467 w472]
            tunnel: w459 -> [w464 _]
            tunnel: [_ w471] -> w458
            tunnel: w457 -> [_ w470]
            tunnel: w456 -> [_ w469]
            tunnel: [_ w468] -> w455
            frame #0 {
              w462 = TRUE  # Last Part of Move?
              n206 = call "3D_Traverse_move.vi"("Mode"=Trav_mode."Read traverse position", "Extra command String"="", "Work in Tunnel Coordinates"=w464, "Home"=Home."Don't Home", "Simulate/Run"=User_Specific_mode."Run VI", "Traverse name"=w467, "Last Part of Move?"=w462) -> ()  [unwired: 10 in, 3 out]
            }
            frame #1 {
              n207 = global read "DriveConfigGlobal.vi" "Configurations"() -> (w473:T22[])
              n208 = for {
                tunnel: w473 -> [w483] mode=indexing
                tunnel: w472 -> [w480]
                shift-right: [w478] -> w471
                shift-left: w470 -> [w479]
                shift-right: [w474] -> w468
                shift-left: w469 -> [w475]
                i -> [w482]
                n209 = Unbundle By Name(w483) -> ("Channel Properties.Metadata Ch Name"=w477:string)
                n210 = Format Into String(format string="%d", initial string=w480, w482) -> (resulting string=w476:string)  [unwired: 1 in, 1 out]
                n211 = Build Array (concatenate)(w479, w477) -> (w478:string[])
                n212 = Build Array (concatenate)(w475, w476) -> (w474:string[])
              }
            }
          }
        }
        n213 = global write "Trav_pos_global.vi" "Traverses to Move"(w444) -> ()
        n214 = global write "Trav_pos_global.vi" "ADAM Positions Ch names"(w445) -> ()
        n215 = global write "Route_mapping_global.vi" "Display Mode"("Display Mode") -> ()
        n216 = global write "Trav_pos_global.vi" "Route checking Chs"(w446) -> ()
      }
      frame "Initialise Measurement Prog" {
        n217 = for {
          tunnel: w507 -> [w518] mode=indexing
          tunnel: [w516] -> w501 mode=concatenating
          n218 = Unbundle By Name(w518) -> ("Meas Setup File"=w517:string)
          n219 = call "Get_array_values_fr_String.vi"("String Value"=w517) -> ("String array"=w516:string[])  [unwired: 1 out]
        }
        n220 = call "Analyse_string_array.vi"("String array"=w501) -> ("Unique strings"=w500:string[])  [unwired: 1 in, 1 out]
        n221 = for {
          tunnel: w500 -> [w511] mode=indexing
          tunnel: [w511] -> w499 mode=indexing if=w510
          n222 = String Subset(string=w511, offset (0)=2, length (rest)=4 ("length (rest)")) -> (substring=w513:string)
          n223 = Not Equal?(x=w513, y="----" ("f")) -> (x != y?=w510:bool)
        }
        n224 = call "Perform_Meas_Setup.vi"("Simulate/Run"=User_Specific_mode."Check VI only", "String array"=w499) -> ("Continue?"=w502:bool)  [unwired: 1 out]
        n225 = Select(t=w505, s=w502, f=Multi_Run_Case."End" ("Multi Run Case")) -> (s? t:f=w504:T3)
      }
      frame "Input Current Position" {
        n226 = call "Save_ADAM_Table_Locally.vi"() -> ()  [unwired: 12 in]
      }
      frame "Experimental setup control" {
        # "#Check- Should this be AND?"
        n227 = global read "Trav_pos_global.vi" "Source Control?"() -> (w527:bool)
        n228 = Or(x=w527, y=w523) -> (x .or. y?=w528:bool)
        n229 = case shown="True" w528 {
          tunnel: w527 -> [_ w531]
          frame False {
          }
          frame True {
            n230 = call "Exp_Setup_Control.vi"("Dispersion?"=w531) -> ()  [unwired: 3 out]
          }
        }
        n231 = global write "Trav_pos_global.vi" "FFID Background"(T6 {"Start X"=0.0, "Start Y"=0.0, "Start Z"=0.0, "End X"=0.0, "End Y"=0.0, "End Z"=0.0, "No. of pts."=0, "Spacing"=enum."Linear", "Filename"=path "", "Tunnel Speed"=0.0, "Averaging time (min)"=0.0, "Extra Commands"="", "Carrier_1 Q (l/min)"=0.0, "Carrier_2 Q (l/min)"=0.0, "Trace Gas Concentration (%)"=0.0, "Specific Arguments"="", "Comments"="", "Row No"=0, "Row Type Selector"=enum."Move Traverse Only", "Completion time"="", "Row Duration (mins)"=0.0, "No. of Valid pts."=0, "Meas Setup File"=""} ("FFID Background")) -> ()
      }
      frame "Check source flowrates" {
        # "#Check- shouldn't we check source flowrates in \"Check\" mode too...?"
        n232 = case shown="\"Run VI\"" w533 {
          tunnel: w534 -> [_ w541]
          frame "Check VI only", Default {
            n233 = Get Date/Time In Seconds() -> (seconds since 1Jan1904=w540:timestamp)
            n234 = global write "Trav_pos_global.vi" "Simulation Time"(w540) -> ()
          }
          frame "Run VI" {
            n235 = for {
              tunnel: w541 -> [w542] mode=indexing
              n236 = call "Set_Source.vi"("Source Status"=Client_Source_Status."Using", "Traverse line"=w542, "Simulate/Run"=User_Specific_mode."Check VI only") -> ()  [unwired: 1 in, 6 out]
            }
          }
        }
        n237 = Increment(x=w538) -> (x+1=w535:T3)
        n238 = Select(t=w538, s=w532, f=w535) -> (s? t:f=w536:T3)
      }
      frame "Setup for running mode" {
        n239 = stacked-sequence {
          seq-local: [_ _ _ _ _ w589 _] -> [_ _ _ _ _ _ w606]
          seq-local: [_ _ _ _ w578 _ _] -> [_ _ _ _ _ w588 _]
          tunnel: w548 -> [w553 _ _ w577 w580 _ _]
          tunnel: w547 -> [_ _ w572 _ _ _ _]
          tunnel: [_ _ _ w575 _ _ _] -> w546
          tunnel: [_ _ _ _ _ w589 _] -> w545
          frame #0 {
            n240 = for {
              tunnel: w553 -> [w557] mode=indexing
              tunnel: [w554] -> w552 mode=indexing
              n241 = Unbundle By Name(w557) -> ("Row Type Selector"=w556:T8)
              n242 = Equal?(x=Multi_run_mode."Synchronize With:" ("Row Type Selector"), y=w556) -> (x = y?=w554:bool)
            }
            n243 = call "Setup_Environment.vi"() -> ()  [unwired: 1 in, 1 out]
            n244 = Or Array Elements(Boolean array=w552) -> (logical OR=w551:bool)
            n245 = case shown="True" w551 {
              frame False {
              }
              frame True {
                n246 = call "Declare_Sync_Client.vi"() -> ()  [unwired: 6 out]
              }
            }
          }
          frame #1 {
            n247 = Open VI Reference(vi path="Display_Trav_Views.vi" ("VI path")) -> (vi reference=w563:refnum<vi>, error out=w562:errorcluster)  [unwired: 1 in, 4 out]
            n248 = global write "Meas_global.vi" "Post Process"(Post_Process."Take New Data" ("Post Process")) -> ()
            n249 = property class="VI"(reference=w563, error in=w562, "Front Panel Window:Open"=FALSE) -> (reference out=w560:refnum<vi>, error out=w559:errorcluster)
            n250 = Close Reference(reference=w560, error in (no error)=w559) -> ()  [unwired: 1 out]
          }
          frame #2 {
            w567 = TRUE  # Start of Multi Run Prog
            w573 = TRUE
            n251 = Get Date/Time In Seconds() -> (seconds since 1Jan1904=w566:timestamp)
            n252 = local read "Command filename"() -> (w571:path)
            n253 = To Double Precision Float(number=w566) -> (double precision float=w565:dbl)
            n254 = global write "Preference_global.vi" "Unblock Email"(w573) -> ()
            n255 = global write "Preference_global.vi" "Unblock SMS"(w573) -> ()
            n256 = global write "Meas_global.vi" "Start Time of experiment"(w565) -> ()
            n257 = Path To String(path=w571) -> (string=w569:string)
            n258 = Concatenate Strings("Commencing a new multi run Prog having the setup filename of :" ("Message"), w569) -> (w568:string)
            n259 = call "Log_Current_row_to_Execute.vi"("Simulate/Run"=w572, "Message"=w568, "Start of Multi Run Prog"=w567) -> ()  [unwired: 2 in, 5 out]
          }
          frame #3 {
            n260 = call "Calc_Remaining_Time.vi"("Currently on Row"=-1, "Table In"=w577) -> ("Estimated Completion time"=w574:string, "Table Out"=w575:T6[])
            n261 = local write "Estimated Completion time"(w574) -> ()
            n262 = global write "Trav_pos_global.vi" "Estimated Completion time"(w574) -> ()
          }
          frame #4 {
            n263 = global read "Trav_pos_global.vi" "Source Control?"() -> (w579:bool)
            n264 = case shown="True" w579 {
              tunnel: w580 -> [_ w584]
              tunnel: [FALSE w582] -> w578
              frame False {
              }
              frame True {
                n265 = for {
                  tunnel: w584 -> [w587] mode=indexing
                  tunnel: [w585] -> w583 mode=indexing
                  n266 = Unbundle By Name(w587) -> ("Trace Gas Concentration (%)"=w586:dbl)
                  n267 = Greater Than 0?(x=w586) -> (x > 0?=w585:bool)
                }
                n268 = Or Array Elements(Boolean array=w583) -> (logical OR=w582:bool)
              }
            }
          }
          frame #5 {
            n269 = case shown="True" w588 {
              tunnel: [TRUE ("T button?") w594] -> w589
              frame False {
              }
              frame True {
                w595 = "EnFlo_Tunnel:Gas Solenoid:Status"
                n270 = Build Array(w595) -> (w598:string[])
                n271 = call "Get_Current_Scan_client.vi"("ADAM Ch Names"=w598) -> ("Numerical Values"=w597:dbl[])  [unwired: 3 out]
                n272 = Index Array(array=w597, index=0) -> (element=w593:dbl)
                n273 = Greater?(x=w593, y=0.5) -> (0:w591:bool)
                n274 = case shown="False" w591 {
                  tunnel: w595 -> [w604 _]
                  tunnel: [w599 TRUE ("T button?")] -> w594
                  frame False {
                    n275 = Format Into String(format string="The \"%s\" ADAM channel is showing that the blue gas button is not on.", w604) -> (resulting string=w602:string)  [unwired: 2 in, 1 out]
                    n276 = Two Button Dialog(message=w602, 1:"Stop" ("F button name (\"Cancel\")"), 2:"Continue" ("T button name (\"OK\")")) -> (T button?=w599:bool)
                  }
                  frame True {
                  }
                }
              }
            }
          }
          frame #6 {
            n277 = case shown="True" w606 {
              frame False {
              }
              frame True {
                n278 = call "Program_Active_Client.vi"("Mode"=enum16{"Program Active", "Traverse Level State"}."Traverse Level State", "Traverse level State"=Traverse_Level_State."Running") -> ()  [unwired: 1 in, 3 out]
              }
            }
          }
        }
      }
      frame "Skip Blank Rows" {
        n279 = stacked-sequence {
          tunnel: w613 -> [w616 w635]
          tunnel: w610 -> [w614 w631]
          frame #0 {
            n280 = Decrement(x=w616) -> (x-1=w615:i32)
            n281 = while {
              tunnel: w614 -> [w626]
              tunnel: w615 -> [w620]
              stop <- w617 continue-if-true
              n282 = local read "Currently on Row"() -> (w622:i32)
              n283 = Increment(x=w622) -> (x+1=w621:i32)
              n284 = Index Array(array=w626, index=w621) -> (element=w625:T6)
              n285 = Less?(x=w621, y=w620) -> (x < y?=w619:bool)
              n286 = Unbundle By Name(w625) -> ("Row Type Selector"=w624:T8)
              n287 = Equal?(x=Multi_run_mode."Blank Row" ("Row Type Selector"), y=w624) -> (x = y?=w618:bool)
              n288 = And(x=w618, y=w619) -> (x .and. y?=w617:bool)
              n289 = case shown="True" w618 {
                tunnel: w621 -> [_ w627]
                frame False {
                }
                frame True {
                  n290 = local write "Currently on Row"(w627) -> ()
                }
              }
            }
          }
          frame #1 {
            n291 = local read "Currently on Row"() -> (w633:i32)
            n292 = Increment(x=w633) -> (x+1=w632:i32)
            n293 = Index Array(array=w631, index=w632) -> (element=w634:T6)
            n294 = Unbundle By Name(w634) -> ("Row Type Selector"=w630:T8)
            n295 = Equal?(x=Multi_run_mode."Turn Off Row Repeating" ("Row Type Selector"), y=w630) -> (x = y?=w628:bool)
            n296 = while {
              shift-right: [w644] -> _
              shift-left: _ -> [w643]
              tunnel: w635 -> [w640]
              tunnel: w633 -> [w644]
              tunnel: w628 -> [w637]
              stop <- TRUE stop-if-true
              n297 = Decrement(x=w640) -> (x-1=w645:i32)
              n298 = Equal?(x=w644, y=w645) -> (x = y?=w638:bool)
              n299 = Not Equal?(x=w644, y=w643) -> (x != y?=w642:bool)
              n300 = Or(x=w637, y=w638) -> (x .or. y?=w636:bool)
              n301 = And(x=w642, y=w636) -> (x .and. y?=w641:bool)
              n302 = case shown="True" w641 {
                tunnel: w640 -> [_ w646]
                frame False {
                }
                frame True {
                  n303 = Initialize Array(timestamp(0 s since 1904-01-01) ("seconds since 1Jan1904"), w646) -> (w648:timestamp[])
                  n304 = global write "Trav_pos_global.vi" "Row completion times"(w648) -> ()
                }
              }
            }
          }
        }
      }
      frame "Which row to execute next" {
        # "last"
        # "Repeat\nRow"
        n305 = local read "Currently on Row"() -> (w649:i32)
        n306 = stacked-sequence {
          seq-local: [_ w678 _] -> [_ _ w715]
          seq-local: [_ w677 _] -> [_ _ w716]
          seq-local: [w658 _ _] -> [_ w676 _]
          seq-local: [_ w673 _] -> [_ _ w709]
          tunnel: [w661 _ _] -> w655
          tunnel: w654 -> [w661 w680 w723]
          tunnel: w653 -> [_ _ w721]
          tunnel: w652 -> [_ w675 w722]
          tunnel: [_ _ w718] -> w651
          tunnel: w650 -> [_ _ w717]
          tunnel: w649 -> [w662 w672 w708]
          frame #0 {
            n307 = Increment(x=w662) -> (x+1=w660:i32)
            n308 = for {
              N: w660 -> [_]
              tunnel: w661 -> [w671] mode=indexing
              shift-right: [w668] -> w658
              shift-left: -1 -> [w665]
              i -> [w666]
              n309 = Unbundle By Name(w671) -> ("Row Type Selector"=w670:T8)
              n310 = Equal?(x=Multi_run_mode."Turn Off Row Repeating" ("Row Type Selector"), y=w670) -> (x = y?=w667:bool)
              n311 = Select(t=w666, s=w667, f=w665) -> (s? t:f=w668:i32)
            }
            n312 = global write "Trav_pos_global.vi" "Currently on point"(0 ("Currently on point")) -> ()
            n313 = global write "Trav_pos_global.vi" "Paused During Row?"(FALSE ("Paused During Row?")) -> ()
          }
          frame #1 {
            n314 = global read "Trav_pos_global.vi" "Row completion times"() -> (w679:timestamp[])
            n315 = global read "Extra_Commands_Global.vi" "Minutes Before Repeating Row"() -> (w674:string)
            n316 = case shown="\"Run VI\"" w675 {
              tunnel: [w681 w682] -> w673
              frame "Check VI only" {
                n317 = global read "Trav_pos_global.vi" "Simulation Time"() -> (w681:timestamp)
              }
              frame "Run VI" {
                n318 = Get Date/Time In Seconds() -> (seconds since 1Jan1904=w682:timestamp)
                n319 = global write "Trav_pos_global.vi" "Simulation Time"(w682) -> ()
              }
            }
            n320 = while {
              tunnel: w680 -> [w693] mode=indexing
              tunnel: w679 -> [w696]
              tunnel: w673 -> [w695]
              tunnel: [w687] -> w678
              tunnel: [w685] -> w677
              tunnel: w676 -> [w684]
              tunnel: w672 -> [w688]
              tunnel: w674 -> [w686]
              i -> [w685]
              stop <- w692 continue-if-true
              n321 = Unbundle By Name(w693) -> ("Extra Commands"=w697:string)
              n322 = call "Extra_Commands.vi"("String to Search"=w697, "Command"=w686) -> ("Numeric Value"=w694:dbl, "Command Found"=w690:bool)  [unwired: 1 in, 3 out]
              n323 = Greater?(x=w685, y=w684) -> (0:w683:bool)
              n324 = And(x=w683, y=w690) -> (x .and. y?=w689:bool)
              n325 = case shown="True" w689 {
                tunnel: w696 -> [_ w703]
                tunnel: w695 -> [_ w704]
                tunnel: w685 -> [_ w702]
                tunnel: w694 -> [_ w700]
                tunnel: [FALSE w699] -> w687
                frame False {
                }
                frame True {
                  n326 = Index Array(array=w703, index=w702) -> (element=w705:timestamp)
                  n327 = Subtract(x=w704, y=w705) -> (x-y=w706:dbl)
                  n328 = Divide(x=w706, y=60.0) -> (x/y=w701:dbl)
                  n329 = Greater?(x=w701, y=w700) -> (0:w699:bool)
                }
              }
              n330 = Less?(x=w685, y=w688) -> (x < y?=w691:bool)
              n331 = Compound Arithmetic op=AND(invert w687, w691) -> (w692:bool)
            }
          }
          frame #2 {
            n332 = Not Equal?(x=w708, y=w716) -> (x != y?=w714:bool)
            n333 = And(x=w715, y=w714) -> (x .and. y?=w713:bool)
            n334 = case shown="True" w713 {
              tunnel: w716 -> [_ w749]
              tunnel: w708 -> [w745 w750]
              tunnel: [w744 w748] -> w719
              tunnel: [w744 w749] -> w710
              tunnel: w721 -> [w747 _]
              tunnel: [w743 TRUE] -> w720
              frame False {
                n335 = Increment(x=w745) -> (x+1=w746:i32)
                n336 = Greater?(x=w747, y=w746) -> (0:w743:bool)
                n337 = Select(t=w746, s=w743, f=w745) -> (s? t:f=w744:i32)
              }
              frame True {
                n338 = Max & Min(x=w750, y=w749) -> (max(x,y)=w748:i32)  [unwired: 1 out]
              }
            }
            n339 = global read "Trav_pos_global.vi" "Row completion times"() -> (w712:timestamp[])
            n340 = case shown="True" w720 {
              tunnel: w710 -> [_ w731]
              tunnel: w723 -> [_ w737]
              tunnel: w722 -> [w725 w729]
              tunnel: w719 -> [_ w735]
              tunnel: [w724 w734] -> w718
              tunnel: w717 -> [_ w734]
              frame False {
                n341 = case shown="\"Run VI\"" w725 {
                  tunnel: [Multi_Run_Case."Show jumped positions" ("Multi Run Case") Multi_Run_Case."Shut down source etc" ("Multi Run Case")] -> w724
                  frame "Check VI only" {
                  }
                  frame "Run VI" {
                  }
                }
              }
              frame True {
                n342 = Index Array(array=w737, index=w731) -> (element=w733:T6)
                n343 = Bundle By Name(cluster=w733, "Row No"=w731) -> (w732:T6)
                n344 = Build Array(w735) -> (w736:i32[])
                n345 = global write "Trav_pos_global.vi" "Meas Setup Number"(0 ("Meas Setup Number")) -> ()
                n346 = property on="Table" class="Arr (strict)"("Index Values"=w736) -> ()  [unwired: 2 in, 2 out]
                n347 = case shown="\"Run VI\"" w729 {
                  selector: w729 -> [_ w739]
                  tunnel: w732 -> [w738 w741]
                  tunnel: [w738 w740] -> w728
                  frame "Check VI only" {
                  }
                  frame "Run VI" {
                    n348 = call "Log_Current_row_to_Execute.vi"("Simulate/Run"=w739, "Start of Multi Run Prog"=FALSE, "Traverse line in"=w741) -> ("Traverse line Out"=w740:T6)  [unwired: 2 in, 4 out]
                  }
                }
                n349 = global write "Trav_pos_global.vi" "Current Row"(w728) -> ()
                "Currently on Row" <- w735
              }
            }
            n350 = Replace Array Subset(array=w712, new element=w709, index=w710) -> (w711:timestamp[])
            n351 = global write "Trav_pos_global.vi" "Row completion times"(w711) -> ()
          }
        }
      }
      frame "Evaluate IF Statement" {
        n352 = global read "Trav_pos_global.vi" "Current Row"() -> (w756:T6)
        n353 = Unbundle By Name(w756) -> ("Extra Commands"=w757:string)
        n354 = global read "Extra_Commands_Global.vi" "If Command"() -> (w760:string)
        n355 = call "Extra_Commands.vi"("String to Search"=w757, "Command"=w760) -> ("String Value"=w759:string, "Command Found"=w753:bool)  [unwired: 1 in, 3 out]
        n356 = And(x=w752, y=w753) -> (x .and. y?=w754:bool)
        n357 = case shown="True" w754 {
          tunnel: w759 -> [_ w770]
          tunnel: [w766 w769] -> w755
          frame False {
            w766 = TRUE  # Execute Row?
          }
          frame True {
            n358 = call "Get_array_values_fr_String.vi"("String Value"=w770) -> ("Numeric Array"=w768:dbl[], "String array"=w767:string[])
            n359 = Index Array(array=w767, index=0 ("Index")) -> (element=w771:string)
            n360 = case shown="\"ADAM Channel Between\"" w771 {
              tunnel: w770 -> [w776 _ _ _]
              tunnel: [w775 w777 w787 TRUE ("Execute Row?")] -> w769
              tunnel: w768 -> [_ w783 w801 _]
              tunnel: w767 -> [_ _ w795 _]
              frame "Time Between" {
                n361 = Get Date/Time In Seconds() -> (seconds since 1Jan1904=w773:timestamp)
                n362 = To Double Precision Float(number=w773) -> (double precision float=w774:dbl)
                n363 = call "If_Time_arguments.vi"("seconds since 1Jan1904"=w774, "String Value"=w776) -> ("Execute Row?"=w775:bool)  [unwired: 2 out]
              }
              frame "Global Value Between" {
                n364 = global read "Extra_Commands_Global.vi" "If command global value"() -> (w778:dbl)
                n365 = Index Array(array=w783, index=1 ("Index")) -> (element=w781:dbl)
                n366 = Index Array(array=w783, index=2 ("Index")) -> (element=w782:dbl)
                n367 = Max & Min(x=w781, y=w782) -> (max(x,y)=w780:dbl, min(x,y)=w779:dbl)
                n368 = In Range and Coerce(upper limit=w780, x=w778, lower limit=w779) -> (In Range?=w777:bool)  [unwired: 1 out]
              }
              frame "ADAM Channel Between" {
                n369 = Index Array(array=w795, index=1 ("Index")) -> (element=w794:string)
                n370 = Build Array(w794) -> (w793:string[])
                n371 = Index Array(array=w801, index=2 ("Index")) -> (element=w799:dbl)
                n372 = Index Array(array=w801, index=3 ("Index")) -> (element=w800:dbl)
                n373 = Max & Min(x=w799, y=w800) -> (max(x,y)=w798:dbl, min(x,y)=w797:dbl)
                n374 = call "Get_Current_Scan_client.vi"("ADAM Ch Names"=w793) -> ("Numerical Values"=w791:dbl[])  [unwired: 3 out]
                n375 = Index Array(array=w791, index=0 ("Index")) -> (element=w790:dbl)
                n376 = In Range and Coerce(upper limit=w798, x=w790, lower limit=w797) -> (In Range?=w788:bool)  [unwired: 1 out]
                n377 = Not A Number/Path/Refnum?(number/path/refnum=w790) -> (NaN/Path/Refnum?=w789:bool)
                n378 = Select(t=TRUE, s=w789, f=w788) -> (s? t:f=w787:bool)
              }
              frame "No Match", Default {
              }
            }
          }
        }
        n379 = Select(t=w763, s=w755, f=Multi_Run_Case."Calculate Row TIme" ("Multi Run Case")) -> (s? t:f=w762:T3)
      }
      frame "Perform Measurement Setup" {
        n380 = global read "Trav_pos_global.vi" "Current Row"() -> (w807:T6)
        n381 = case shown="\"Run VI\"" w806 {
          selector: w806 -> [_ w811]
          tunnel: w807 -> [_ w812]
          frame "Check VI only" {
          }
          frame "Run VI" {
            n382 = stacked-sequence {
              tunnel: w812 -> [w815 _]
              tunnel: w811 -> [w813 _]
              frame #0 {
                n383 = Unbundle By Name(w815) -> ("Extra Commands"=w814:string)
                n384 = call "Pause_for_server_ch_val.vi"("Extra command string"=w814, "Simulate/Run"=w813) -> ()  [unwired: 2 out]
              }
              frame #1 {
                n385 = Get Date/Time In Seconds() -> (seconds since 1Jan1904=w816:timestamp)
                n386 = To Double Precision Float(number=w816) -> (double precision float=w817:dbl)
                n387 = global write "Trav_pos_global.vi" "Start of Row time (Sec)"(w817) -> ()
              }
            }
          }
        }
      }
      frame "Set Measurement Conditions" {
        w823 = TRUE  # Row Completed
        w822 = FALSE  # Row Completed
        n388 = global read "Trav_pos_global.vi" "Current Row"() -> (w820:T6)
        n389 = Unbundle By Name(w820) -> ("Row Type Selector"=w825:T8)
        n390 = case shown="\"Send Message\"" w825 {
          tunnel: [TRUE FALSE TRUE TRUE TRUE TRUE FALSE TRUE FALSE w874 FALSE FALSE FALSE] -> w830
          tunnel: w820 -> [w838 w841 w844 w847 w850 w853 w856 w859 w868 w873 w895 w898 w901]
          tunnel: [w838 w841 w844 w847 w850 w853 w856 w859 w867 w872 w895 w898 w901] -> w826
          tunnel: [w837 w840 w843 w846 w849 w852 w855 w858 w863 w871 w894 w897 w900] -> w824
          tunnel: w823 -> [w837 _ w843 w846 w849 _ _ _ _ w871 w894 w897 w900]
          tunnel: w822 -> [_ w840 _ _ _ w852 w855 w858 w863 _ _ _ _]
          tunnel: w818 -> [_ _ _ _ _ _ _ _ _ w870 _ _ _]
          frame "Move Traverse Only" {
          }
          frame "Check Beam Power" {
          }
          frame "Set Tunnel Speed Only" {
          }
          frame "Set Source Only" {
          }
          frame "Set Measurement Conditions" {
          }
          frame "Single Measurement" {
          }
          frame "Vertical Profile", Default {
          }
          frame "Scanning Valve Measurement" {
          }
          frame "Run VI Named:" {
            n391 = global read "Extra_Commands_Global.vi" "Skip Source Demand"() -> (w866:string)
            n392 = global read "Extra_Commands_Global.vi" "Establish Exp Conditions (s)"() -> (w862:string)
            n393 = Unbundle By Name(w868) -> ("Extra Commands"=w865:string)
            n394 = Concatenate Strings(w862, " = 0" ("Substring"), w866, w865) -> (w864:string)
            n395 = Bundle By Name(cluster=w868, "Extra Commands"=w864) -> (w867:T6)
          }
          frame "Send Message" {
            n396 = stacked-sequence {
              tunnel: [_ _ FALSE] -> w874
              tunnel: w873 -> [w882 w888 w891]
              tunnel: [_ _ w891] -> w872
              tunnel: w870 -> [w875 _ _]
              frame #0 {
                n397 = Unbundle By Name(w882) -> ("Specific Arguments"=w877:string, "Comments"=w878:string, "Filename"=w880:path)
                n398 = Concatenate Strings(w877, w878) -> (w876:string)
                n399 = Build Array(w880) -> (w879:path[])
                n400 = case shown="\"Run VI\"" w875 {
                  tunnel: "Message" ("Error Type") -> [_ w885]
                  tunnel: w876 -> [_ w884]
                  tunnel: w879 -> [_ w883]
                  frame "Check VI only", Default {
                  }
                  frame "Run VI" {
                    n401 = call "Email_Text_Files.vi"("Filenames"=w883, "message"=w884, "subject ([No Subject])"=w885) -> ()
                  }
                }
              }
              frame #1 {
                n402 = Unbundle By Name(w888) -> ("Extra Commands"=w889:string)
                n403 = global read "Extra_Commands_Global.vi" "Establish Exp Conditions (s)"() -> (w890:string)
                n404 = call "Extra_Commands.vi"("String to Search"=w889, "Command"=w890) -> ("Numeric Value"=w886:dbl)  [unwired: 1 in, 4 out]
                n405 = call "Wait_Seconds_with_display.vi"("Message"="In Send Message Row", "Seconds to wait"=w886) -> ()  [unwired: 2 out]
              }
              frame #2 {
              }
            }
          }
          frame "Fall Back to this Row" {
          }
          frame "Turn Off Row Repeating" {
          }
          frame "Blank Row" {
          }
        }
        n406 = case shown="True" w830 {
          tunnel: w826 -> [_ w903]
          tunnel: w818 -> [_ w907]
          tunnel: [Multi_Run_Status."Continue" ("Status") w904] -> w819
          frame False {
          }
          frame True {
            w906 = 1  # Currently on Point
            n407 = call "Program_Active.vi"() -> ()  [unwired: 1 in]
            n408 = call "Set_Measurement_Conditions.vi"("Simulate/Run"=w907, "Currently on Point"=w906, "Traverse line"=w903) -> ("Status Cluster"=w905:T25)  [unwired: 2 out]
            n409 = Unbundle By Name(w905) -> ("Status"=w904:T2)
          }
        }
        n410 = case shown="\"Continue\"" w819 {
          tunnel: [w834 Multi_Run_Case."Calculate Row TIme" ("Multi Run Case")] -> w829
          tunnel: w828 -> [w835 _]
          tunnel: w824 -> [w832 _]
          frame "Continue" {
            n411 = Select(t=Multi_Run_Case."Calculate Row TIme" ("Multi Run Case"), s=w832, f=w835) -> (s? t:f=w834:T3)
          }
          frame "Jump to Next Point", Default {
          }
        }
        n412 = local write "Status"(w819) -> ()
      }
      frame "Execute Row" {
        n413 = global read "Trav_pos_global.vi" "Current Row"() -> (w909:T6)
        n414 = stacked-sequence {
          tunnel: w910 -> [w914 w925 w927]
          tunnel: w909 -> [w915 w922 w926]
          frame #0 {
            n415 = case shown="\"Check VI only\"" w914 {
              selector: w914 -> [w916 _]
              tunnel: w915 -> [w918 _]
              frame "Check VI only" {
                n416 = Unbundle By Name(w918) -> ("Extra Commands"=w919:string, "Row No"=w921:i32, "Meas Setup File"=w917:string)
                n417 = call "Skip_If Sd_Error_Below.vi"("String to Search"=w919, "Simulate/Run"=w916, "Measurement setup Applied?"=TRUE, "Row Number"=w921, "Measurement Setup File"=w917) -> ()  [unwired: 5 out]
              }
              frame "Run VI" {
              }
            }
          }
          frame #1 {
            n418 = call "Execute_Row.vi"("Simulate/Run"=w925, "Traverse line"=w922) -> ("Status"=w924:T2, "Traverse line out"=w923:T6)  [unwired: 2 out]
            n419 = local write "Status"(w924) -> ()
            n420 = global write "Trav_pos_global.vi" "Current Row"(w923) -> ()
          }
          frame #2 {
            w930 = FALSE  # Empty list
            n421 = call "Remember_RD_Folders.vi"("Empty list"=w930) -> ("List of Folders"=w929:path[])  [unwired: 1 in]
            n422 = for {
              tunnel: w926 -> [w935]
              tunnel: w929 -> [w934] mode=indexing
              tunnel: "Muti_Run_Log.xls" ("name or relative path") -> [w932]
              tunnel: w927 -> [w931]
              n423 = Build Path(base path=w934, name or relative path=w932) -> (appended path=w933:path)
              n424 = call "Log_Current_row_to_Execute.vi"("Simulate/Run"=w931, "Start of Multi Run Prog"=FALSE, "Traverse line in"=w935, "Multi Run Log File"=w933) -> ()  [unwired: 1 in, 5 out]
            }
          }
        }
      }
      frame "Calculate Row TIme" {
        n425 = global read "Trav_pos_global.vi" "Paused During Row?"() -> (w941:bool)
        n426 = local read "Status"() -> (w943:T2)
        n427 = global read "Trav_pos_global.vi" "Current Row"() -> (w940:T6)
        n428 = Equal?(x=w943, y=Multi_Run_Status."Continue" ("Status")) -> (x = y?=w942:bool)
        n429 = Compound Arithmetic op=AND(w942, w937, invert w941) -> (w939:bool)
        n430 = case shown="False" w939 {
          tunnel: w940 -> [w956 w967]
          frame False {
            n431 = global read "Trav_pos_global.vi" "Simulation Time"() -> (w957:timestamp)
            n432 = To Double Precision Float(number=w957) -> (double precision float=w951:dbl)
            n433 = call "Calculate_Row_Time.vi"("Row Start Time (Sec Since 1904)"=w951, "Multi Run Row"=w956) -> ("Scalable Time (Sec)"=w954:dbl, "Fixed Time (Sec)"=w952:dbl)
            n434 = call "Overhead_Factor.vi"("Mode"=Overhead."Read Current Overhead") -> ("Current Overhead Factor"=w955:dbl)  [unwired: 3 in]
            n435 = Multiply(x=w954, y=w955) -> (x*y=w953:dbl)
            n436 = Add(x=w952, y=w953) -> (x+y=w948:dbl)
            n437 = Add(x=w951, y=w948) -> (x+y=w950:dbl)
            n438 = global write "Trav_pos_global.vi" "Start of Row time (Sec)"(w948) -> ()
            n439 = To Time Stamp(1:w950) -> (0:w949:timestamp)
            n440 = global write "Trav_pos_global.vi" "Simulation Time"(w949) -> ()
          }
          frame True {
            n441 = global read "Trav_pos_global.vi" "Start of Row time (Sec)"() -> (w965:dbl)
            n442 = Get Date/Time In Seconds() -> (seconds since 1Jan1904=w960:timestamp)
            n443 = To Double Precision Float(number=w960) -> (double precision float=w959:dbl)
            n444 = call "Calculate_Row_Time.vi"("Row Start Time (Sec Since 1904)"=w965, "Multi Run Row"=w967) -> ("Scalable Time (Sec)"=w961:dbl, "Fixed Time (Sec)"=w963:dbl)
            n445 = Subtract(x=w959, y=w965) -> (x-y=w964:dbl)
            n446 = Subtract(x=w964, y=w963) -> (x-y=w962:dbl)
            n447 = call "Overhead_Factor.vi"("Sum of Ideal times (Sec)"=w961, "Sum of Actual times (Sec)"=w962, "Mode"=Overhead."Update total times") -> ()  [unwired: 1 in, 1 out]
          }
        }
      }
      frame "Update time estimate" {
        n448 = global read "Trav_pos_global.vi" "Current Row"() -> (w971:T6)
        n449 = local read "Currently on Row"() -> (w970:i32)
        n450 = Unbundle By Name(w971) -> ("Row No"=w969:i32)
        n451 = Equal?(x=w969, y=w970) -> (x = y?=w968:bool)
        n452 = case shown="\"Run VI\"" w974 {
          tunnel: w977 -> [w980 w1008]
          tunnel: [w985 w1004] -> w976
          tunnel: w973 -> [_ w1010]
          tunnel: [w984 w1009] -> w972
          tunnel: w970 -> [w982 w1003]
          tunnel: w971 -> [w983 w1007]
          tunnel: w968 -> [w981 w1006]
          frame "Check VI only" {
            n453 = global read "Trav_pos_global.vi" "Simulation Time"() -> (w987:timestamp)
            n454 = To Double Precision Float(number=w987) -> (double precision float=w986:dbl)
            n455 = call "Sec_to_date_filename.vi"("seconds"=w986) -> ("Day"=w989:string, "Time"=w988:string)  [unwired: 2 out]
            n456 = Concatenate Strings(w988, "  " ("Substring"), w989) -> (w984:string)
            n457 = case shown="True" w981 {
              tunnel: w982 -> [_ w1000]
              tunnel: [w991 w998] -> w985
              tunnel: w984 -> [_ w997]
              tunnel: w983 -> [_ w996]
              tunnel: w980 -> [w991 w992]
              frame False {
              }
              frame True {
                n458 = global read "Trav_pos_global.vi" "Start of Row time (Sec)"() -> (w995:dbl)
                n459 = Divide(x=w995, y=60.0) -> (x/y=w993:dbl)
                n460 = Bundle By Name(cluster=w996, "Completion time"=w997, "Row Duration (mins)"=w993) -> (w999:T6)
                n461 = Replace Array Subset(array=w992, new element=w999, index=w1000) -> (w998:T6[])
              }
            }
          }
          frame "Run VI" {
            n462 = case shown="True" w1006 {
              tunnel: w1003 -> [_ w1017]
              tunnel: w1008 -> [w1013 w1016]
              tunnel: w1007 -> [_ w1015]
              tunnel: [w1013 w1014] -> w1005
              frame False {
              }
              frame True {
                n463 = Replace Array Subset(array=w1016, new element=w1015, index=w1017) -> (w1014:T6[])
              }
            }
            n464 = Decrement(x=w1010) -> (x-1=w1012:i32)
            n465 = call "Calc_Remaining_Time.vi"("Currently on Row"=w1003, "Table In"=w1005) -> ("Table Out"=w1004:T6[])  [unwired: 1 out]
            n466 = Index Array(array=w1004, index=w1012) -> (element=w1011:T6)
            n467 = Unbundle By Name(w1011) -> ("Completion time"=w1009:string)
            n468 = call "Program_Active_Client.vi"("Mode"=enum16{"Program Active", "Traverse Level State"}."Traverse Level State", "Traverse level State"=Traverse_Level_State."Running") -> ()  [unwired: 1 in, 3 out]
          }
        }
        "Estimated Completion time" <- w972
        n469 = global write "Trav_pos_global.vi" "Estimated Completion time"(w972) -> ()
      }
      frame "Pause Multi Run Program" {
        n470 = while {
          tunnel: "Pause" -> [w1029]
          tunnel: [w1032] -> w1024
          tunnel: w1023 -> [w1031]
          tunnel: w1021 -> [w1030]
          shift-right: [w1029] -> _
          shift-left: _ -> [w1028]
          stop <- TRUE stop-if-true
          n471 = case shown="True" w1029 {
            selector: w1029 -> [_ w1034]
            tunnel: [w1033 w1038] -> w1032
            tunnel: w1031 -> [w1033 w1036]
            tunnel: w1030 -> [_ w1037]
            tunnel: w1028 -> [_ w1035]
            frame False {
            }
            frame True {
              n472 = stacked-sequence {
                tunnel: w1036 -> [_ _ _ _ w1053]
                tunnel: [_ _ _ _ w1054] -> w1038
                tunnel: w1037 -> [w1040 _ _ _ _]
                tunnel: w1034 -> [_ _ _ w1049 _]
                tunnel: w1035 -> [_ _ _ w1048 _]
                frame #0 {
                  n473 = Quotient & Remainder(x=w1040, y=15) -> (x-y*floor(x/y)=w1039:i32)  [unwired: 1 out]
                  n474 = case shown="0" w1039 {
                    frame 0 {
                      n475 = Current VI's Path() -> (path=w1042:path)
                      n476 = call "Bring_to_front.vi"("path"=w1042) -> ()
                    }
                    frame 1, Default {
                    }
                  }
                }
                frame #1 {
                  n477 = global write "Trav_pos_global.vi" "Paused During Row?"(TRUE ("Paused During Row?")) -> ()
                  "Pause message" <- "Multi Run Program Paused!!!!" ("Pause message")
                }
                frame #2 {
                  n478 = property on="Pause message" class="Str"("Visible"=TRUE) -> ()  [unwired: 2 in, 2 out]
                  n479 = Wait Until Next ms Multiple(millisecond multiple=u32 1500) -> ()  [unwired: 1 out]
                }
                frame #3 {
                  n480 = Compound Arithmetic op=AND(w1049, invert w1048) -> (w1047:bool)
                  n481 = case shown="True" w1047 {
                    frame False {
                    }
                    frame True {
                      n482 = call "Program_Active_Client.vi"("Mode"=enum16{"Program Active", "Traverse Level State"}."Program Active", "Time till next contact (Sec)"=12000.0, "Traverse level State"=Traverse_Level_State."Running") -> ()  [unwired: 3 out]
                    }
                  }
                }
                frame #4 {
                  n483 = property on="Pause message" class="Str"("Visible"=FALSE) -> ()  [unwired: 2 in, 2 out]
                  n484 = Wait Until Next ms Multiple(millisecond multiple=u32 1500) -> ()  [unwired: 1 out]
                  n485 = Decrement(x=w1053) -> (x-1=w1054:T3)
                }
              }
            }
          }
        }
        n486 = call "Overhead_Factor.vi"("Mode"=Overhead."Read Current Overhead") -> ("Current Overhead Factor"=→"Current Overhead Factor":dbl)  [unwired: 3 in]
      }
      frame "Do Another Row?" {
        w1066 = Multi_Run_Status."Terminate Run" ("Status")
        n487 = global read "Preference_global.vi" "Server Comms"() -> (w1061:T26)
        n488 = case shown="\"Server Link Healthy\"" w1061 {
          tunnel: [w1075 TRUE] -> w1060
          frame "Server Link Healthy" {
            n489 = Build Array("EnFlo Lab:Emergency_Stop:Happy") -> (w1078:string[])
            n490 = call "Get_Current_Scan_client.vi"("ADAM Ch Names"=w1078) -> ("Numerical Values"=w1080:dbl[])  [unwired: 1 in, 2 out]
            n491 = Index Array(array=w1080) -> (element=w1076:dbl)  [unwired: 1 in]
            n492 = Not A Number/Path/Refnum?(number/path/refnum=w1076) -> (NaN/Path/Refnum?=w1077:bool)
            n493 = case shown="True" w1077 {
              tunnel: w1076 -> [w1083 _]
              tunnel: [w1081 TRUE] -> w1075
              frame False {
                n494 = Greater?(x=w1083, y=0.5) -> (0:w1081:bool)
              }
              frame True {
              }
            }
          }
          frame "Do Not Link To Server" {
          }
        }
        n495 = case shown="False" "Stop after Repeats" {
          tunnel: w1062 -> [_ w1089]
          frame False {
            n496 = local read "Currently on Row"() -> (w1087:i32)
            n497 = Increment(x=w1087) -> (x+1=→"Last Row Run":i32)
          }
          frame True {
            n498 = Decrement(x=w1089) -> (x-1=w1088:i32)
            n499 = local write "Currently on Row"(w1088) -> ()
          }
        }
        n500 = case shown="True" "stop" {
          tunnel: [w1090 w1091] -> w1067
          tunnel: w1066 -> [_ w1091]
          frame False {
            n501 = local read "Status"() -> (w1090:T2)
          }
          frame True {
            n502 = local write "Status"(w1091) -> ()
          }
        }
        n503 = Not Equal?(x=w1066, y=w1067) -> (x != y?=w1065:bool)
        n504 = case shown="True" w1065 {
          tunnel: [w1092 w1096] -> w1058
          tunnel: w1070 -> [w1093 _]
          tunnel: w1067 -> [_ w1097]
          frame False {
            n505 = case shown="\"Run VI\"" w1093 {
              tunnel: [Multi_Run_Case."Show jumped positions" ("Multi Run Case") Multi_Run_Case."Shut down source etc" ("Multi Run Case")] -> w1092
              frame "Check VI only" {
              }
              frame "Run VI" {
              }
            }
          }
          frame True {
            n506 = case shown="\"Jump To Fall Back\"" w1097 {
              tunnel: [Multi_Run_Case."Skip Blank Rows" ("Multi Run Case") Multi_Run_Case."Find Next Fall Back Row" ("Multi Run Case")] -> w1096
              frame "Continue", Default {
              }
              frame "Jump To Fall Back" {
              }
            }
          }
        }
        n507 = local read "Display Mode"() -> (w1057:T5)
        n508 = case shown="False" w1060 {
          tunnel: [Multi_Run_Case."Shut down source etc" ("Multi Run Case") w1074] -> w1059
          tunnel: w1058 -> [_ w1074]
          frame False {
            n509 = local write "Status"(Multi_Run_Status."Terminate Run" ("Status")) -> ()
          }
          frame True {
          }
        }
        n510 = global write "Route_mapping_global.vi" "Display Mode"(w1057) -> ()
      }
      frame "Find Next Fall Back Row" {
        n511 = local read "Currently on Row"() -> (w1102:i32)
        n512 = Increment(x=w1102) -> (x+1=w1101:i32)
        n513 = Greater?(x=w1100, y=w1101) -> (0:w1108:bool)
        n514 = Index Array(array=w1109, index=w1102) -> (element=w1110:T6)
        n515 = Unbundle By Name(w1110) -> ("Row Type Selector"=w1105:T8)
        n516 = Equal?(x=w1105, y=Multi_run_mode."Fall Back to this Row" ("Mode")) -> (x = y?=w1103:bool)
        n517 = case shown="True" w1108 {
          tunnel: [Multi_Run_Case."Skip Blank Rows" ("Multi Run Case") w1117] -> w1107
          tunnel: w1103 -> [_ w1113]
          tunnel: w1102 -> [_ w1114]
          frame False {
          }
          frame True {
            n518 = case shown="False" w1113 {
              tunnel: w1114 -> [w1119 _]
              frame False {
                n519 = Increment(x=w1119) -> (x+1=w1118:i32)
                n520 = local write "Currently on Row"(w1118) -> ()
              }
              frame True {
              }
            }
            n521 = Select(t=Multi_Run_Case."Skip Blank Rows" ("Multi Run Case"), s=w1113, f=Multi_Run_Case."Find Next Fall Back Row" ("Multi Run Case")) -> (s? t:f=w1117:T3)
          }
        }
      }
      frame "Shut down source etc" {
        n522 = for {
          tunnel: w1138 -> [w1160] mode=indexing
          tunnel: Multi_run_mode."Synchronize With:" ("Mode") -> [w1158]
          tunnel: [w1157] -> w1140 mode=indexing
          n523 = Unbundle By Name(w1160) -> ("Row Type Selector"=w1159:T8)
          n524 = Equal?(x=w1159, y=w1158) -> (x = y?=w1157:bool)
        }
        n525 = call "Program_Active_Client.vi"("Mode"=enum16{"Program Active", "Traverse Level State"}."Traverse Level State", "Traverse level State"=Traverse_Level_State."Complete") -> ()  [unwired: 1 in, 3 out]
        n526 = call "Overhead_Factor.vi"("Mode"=Overhead."Re Scale totals to 3 hrs") -> ()  [unwired: 3 in, 1 out]
        n527 = local read "Status"() -> (w1128:T2)
        n528 = global read "Trav_pos_global.vi" "Source Control?"() -> (w1120:bool)
        n529 = global read "Meas_global.vi" "Start Time of experiment"() -> (w1136:dbl)
        n530 = Equal?(x=w1128, y=Multi_Run_Status."Terminate Run" ("Status")) -> (x = y?=w1126:bool)
        n531 = Or Array Elements(Boolean array=w1140) -> (logical OR=w1129:bool)
        n532 = Compound Arithmetic op=AND(w1129, invert w1126) -> (w1130:bool)
        n533 = Get Date/Time In Seconds() -> (seconds since 1Jan1904=w1121:timestamp)
        n534 = case shown="True" w1130 {
          frame False {
          }
          frame True {
            n535 = global read "Preference_global.vi" "Rig Setup"() -> (w1150:string)
            n536 = Concatenate Strings(w1150, ":Program:Sync") -> (w1152:string)
            n537 = Bundle By Name(cluster=T20 {"Channel Name"="", "New Value"=0.0} ("Update Scan Value Cluster"), "Channel Name"=w1152, "New Value"=1000.0 ("Bundle Element")) -> (w1153:T20)
            n538 = Build Array(w1153) -> (w1155:T20[])
            n539 = call "Update_Current_Value_client.vi"("Update array in"=w1155) -> ()  [unwired: 1 in]
          }
        }
        n540 = case shown="True" w1120 {
          frame False {
          }
          frame True {
            w1148 = u32 1  # Time to hold source OFF (microseconds)
            w1149 = u32 0  # Time to hold source ON (microseconds)
            n541 = call "Set_Source.vi"("Source Status"=Client_Source_Status."Not Using", "Simulate/Run"=User_Specific_mode."Run VI") -> ()  [unwired: 2 in, 6 out]
            n542 = call "Arduino_Timed_Release.vi"("Time to hold source ON (microseconds)"=w1149, "Time to hold source OFF (microseconds)"=w1148, "Number of cycles"=u16 1) -> ()  [unwired: 2 out]
          }
        }
        n543 = To Double Precision Float(number=w1121) -> (double precision float=w1137:dbl)
        n544 = Subtract(x=w1137, y=w1136) -> (x-y=w1135:dbl)
        n545 = Greater?(x=w1135, y=300.0) -> (0:w1132:bool)
        n546 = Not(x=w1132) -> (.not. x?=→"Non Starter":bool)
        n547 = Increment(x=w1124) -> (x+1=w1123:T3)
        n548 = Increment(x=w1123) -> (x+1=w1122:T3)
        n549 = Select(t=w1124, s=w1132, f=w1122) -> (s? t:f=w1133:T3)
      }
      frame "Email results to users" {
        n550 = local read "Currently on Row"() -> (w1166:i32)
        n551 = Increment(x=w1166) -> (x+1=w1161:i32)
        n552 = Split 1D Array(array=w1163, index=w1161) -> (first subarray=w1170:T6[], second subarray=w1169:T6[])
        n553 = Array Size(array=w1169) -> (size(s)=w1171:i32)
        n554 = for {
          tunnel: w1170 -> [w1186] mode=indexing
          shift-right: [w1184] -> w1172
          shift-left: string[] [] -> [w1185]
          n555 = Unbundle By Name(w1186) -> ("Row Type Selector"=w1177:T8, "Filename"=w1183:path, "Comments"=w1182:string)
          n556 = Not Equal?(x=Multi_run_mode."Auto Calibrate" ("Row Type Selector"), y=w1177) -> (x != y?=w1179:bool)
          n557 = Empty String/Path?(string/path=w1183) -> (empty?=w1180:bool)
          n558 = Compound Arithmetic op=AND(w1179, invert w1180) -> (w1178:bool)
          n559 = case shown="True" w1178 {
            tunnel: w1185 -> [w1187 w1195]
            tunnel: [w1187 w1194] -> w1184
            tunnel: w1183 -> [_ w1193]
            tunnel: w1182 -> [_ w1191]
            frame False {
            }
            frame True {
              n560 = Path To String(path=w1193) -> (string=w1192:string)
              n561 = Match Pattern(string=w1191, regular expression=" !!Program added comments") -> (after substring=w1188:string)  [unwired: 4 out]
              n562 = Concatenate Strings(w1192, w1188) -> (w1190:string)
              n563 = Build Array (concatenate)(w1195, w1190) -> (w1194:string[])
            }
          }
        }
        n564 = Equal To 0?(x=w1171) -> (x = 0?=w1162:bool)
        n565 = case shown="False" w1162 {
          tunnel: ["Having completed only some of the requested rows." ("Message") ""] -> w1167
          frame False {
          }
          frame True {
          }
        }
        n566 = call "End_of_run_messages.vi"("Message"=w1167, "Subject"="Multi Run Ended", "Attachments"=w1172) -> ()  [unwired: 1 in]
      }
      frame "Save run efficiency" {
        w1209 = FALSE  # append to file? (new file:F)
        w1208 = FALSE  # advisory dialog? (display:T)
        n567 = call "Get_IP_Number.vi"() -> ("Computer Name"=w1197:string)  [unwired: 1 out]
        n568 = Format Into String(format string="Preferences_%s.xls" ("name or relative path"), w1197) -> (resulting string=w1196:string)  [unwired: 2 in, 1 out]
        n569 = call "Setup_Filepath.vi"("Setup File Type"=Setup_Filetype."General", "Filename in"=w1196) -> ("Filename Out"=w1199:path)  [unwired: 1 out]
        n570 = call "Overhead_Factor.vi"("Mode"=Overhead."Read Current Overhead") -> ("Current Overhead Factor"=w1203:dbl)  [unwired: 3 in]
        n571 = Number To Fractional String(number=w1203, precision (6)=i16 4) -> (F-format string=w1201:string)  [unwired: 2 out]
        n572 = call "Read_Characters_From_File.ph.vi"("file path (dialog if empty)"=w1199) -> ("character string"=w1206:string)  [unwired: 1 in, 7 out]
        n573 = call "Replace_data_in_setup_string.vi"("New data string"=w1201, "Input string"=w1206, "Variable name"="Current Overhead Factor") -> ("Appended string"=w1205:string)
        n574 = call "Write_Characters_To_File.vi"("file path (dialog if empty)"=w1199, "advisory dialog? (display:T)"=w1208, "character string"=w1205, "append to file? (new file:F)"=w1209) -> ()  [unwired: 1 in, 4 out]
      }
      frame "Remove Skipped Commands" {
        n575 = for {
          tunnel: w1215 -> [w1223] mode=indexing
          tunnel: [w1222] -> w1214 mode=indexing
          n576 = Unbundle By Name(w1223) -> ("Comments"=w1221:string)
          n577 = Match Pattern(string=w1221, regular expression=" !!Program added comments") -> (before substring=w1220:string)  [unwired: 4 out]
          n578 = Bundle By Name(cluster=w1223, "Comments"=w1220) -> (w1222:T6)
        }
      }
      frame "Show jumped positions" {
        n579 = global read "Trav_pos_global.vi" "Jumped Positions"() -> (w1226:dbl[][])
        n580 = Array Size(array=w1226) -> (size(s)=w1229:i32[])
        n581 = Index Array(array=w1229, index=0) -> (element=w1225:i32)
        n582 = Greater Than 0?(x=w1225) -> (x > 0?=w1227:bool)
        n583 = case shown="True" w1227 {
          tunnel: w1226 -> [_ w1240]
          tunnel: w1225 -> [_ w1239]
          frame False {
            n584 = Current VI's Path() -> (path=w1234:path)
            n585 = Open VI Reference(vi path=w1234) -> (vi reference=w1235:refnum<vi>, error out=w1236:errorcluster)  [unwired: 1 in, 4 out]
            n586 = property class="VI"(reference=w1235, error in=w1236, "Front Panel Window:Is Frontmost"=TRUE) -> (reference out=w1237:refnum<vi>, error out=w1238:errorcluster)
            n587 = Close Reference(reference=w1237, error in (no error)=w1238) -> ()  [unwired: 1 out]
          }
          frame True {
            n588 = stacked-sequence {
              tunnel: w1240 -> [w1241 w1251]
              tunnel: w1239 -> [w1245 _]
              frame #0 {
                w1246 = TRUE  # Open Front Panel
                w1247 = FALSE  # Crash?
                n589 = global read "Trav_pos_global.vi" "Default Traverse Setup"() -> (w1242:string)
                n590 = Format Into String(format string="There are %d points which cannot be reached", w1245) -> (resulting string=w1243:string)  [unwired: 2 in, 1 out]
                n591 = call "Display_Trav_Views.vi"("Current Probe Position"=w1241, "Traverse Name"=w1242, "Open Front Panel"=w1246, "Error Comments"=w1243, "Crash?"=w1247) -> ()  [unwired: 2 in, 4 out]
              }
              frame #1 {
                n592 = local read "Command filename"() -> (w1255:path)
                n593 = Array To Spreadsheet String(array=w1251, 3:"%.1f" ("format string")) -> (spreadsheet string=w1249:string)  [unwired: 1 out]
                n594 = Strip Path(path=w1255) -> (stripped path=w1254:path)  [unwired: 1 out]
                n595 = Build Path(base path=w1254, name or relative path="Jumped_Positions.xls") -> (appended path=w1252:path)
                n596 = call "Write_File_Simple.vi"("append to file? (new file:F)"=FALSE, "character string"=w1249, "file path"=w1252) -> ()  [unwired: 2 out]
              }
            }
          }
        }
      }
      frame "Save Setup to File" {
        w1275 = FALSE  # Start of Multi Run Prog
        n597 = local read "Status"() -> (w1270:T2)
        n598 = local read "Command filename"() -> (w1262:path)
        n599 = local read "Stop after Repeats"() -> (w1273:bool)
        n600 = local read "Last Row Run"() -> (w1258:i32)
        n601 = local read "stop"() -> (w1274:bool)
        n602 = local read "Non Starter"() -> (w1256:bool)
        n603 = Equal?(x=w1270, y=Multi_Run_Status."Continue" ("Status")) -> (x = y?=w1269:bool)
        n604 = Less?(x=w1268, y=T9."Run Multi Run Prog") -> (x < y?=w1257:bool)
        n605 = Decrement(x=w1258) -> (x-1=w1266:i32)
        n606 = Equal?(x=w1259, y=w1258) -> (x = y?=w1282:bool)
        n607 = Equal To 0?(x=w1258) -> (x = 0?=w1281:bool)
        n608 = Compound Arithmetic op=OR(w1273, w1274, w1269) -> (w1272:bool)
        n609 = Select(t=w1258, s=w1272, f=w1266) -> (s? t:f=w1276:i32)
        n610 = call "Current_Filepath.vi"("Short_Name"="Cmd" ("Data Type"), "Filename in"=w1262, "Data Type"="Commands") -> ("Filename Out"=w1261:path)  [unwired: 1 in, 1 out]
        n611 = Compound Arithmetic op=OR(w1282, w1281, w1257, w1256) -> (w1283:bool)
        n612 = Split 1D Array(array=w1287, index=w1276) -> (second subarray=w1290:T6[])  [unwired: 1 out]
        n613 = local read "Work in Tunnel Coordinates?"() -> (w1265:T1)
        n614 = Path To String(path=w1261) -> (string=w1280:string)
        n615 = local read "Jump Bad Positions"() -> (w1264:bool)
        n616 = case shown="False" w1283 {
          tunnel: w1261 -> [w1299 w1333]
          tunnel: [w1298 w1333] -> w1291
          tunnel: w1290 -> [w1296 _]
          tunnel: [w1295 w1334] -> w1289
          tunnel: w1287 -> [w1297 w1334]
          tunnel: w1265 -> [w1294 _]
          tunnel: w1264 -> [w1293 _]
          frame False {
            n617 = stacked-sequence {
              tunnel: w1299 -> [w1301 w1312 _]
              tunnel: [_ w1305 _] -> w1298
              tunnel: w1297 -> [w1304 _ w1317]
              tunnel: w1296 -> [_ _ w1315]
              tunnel: [_ _ w1314] -> w1295
              tunnel: w1294 -> [w1303 _ _]
              tunnel: w1293 -> [w1302 _ _]
              frame #0 {
                n618 = global write "Trav_pos_global.vi" "Sync to server now"(TRUE) -> ()
                n619 = call "Save_Trav_setup.vi"("Work in Tunnel Coordinates?"=w1303, "Trav Table"=w1304, "Jump Bad Positions"=w1302, "Setup filename"=w1301) -> ()  [unwired: 2 out]
              }
              frame #1 {
                n620 = Strip Path(path=w1312) -> (stripped path=w1313:path, name=w1311:string)
                n621 = call "Add_filename_suffix.vi"("Filename"=w1311) -> ("Original Suffix"=w1308:string, "Base name"=w1310:string)  [unwired: 1 in, 2 out]
                n622 = Concatenate Strings(w1310, "_Rem", w1308) -> (w1307:string)
                n623 = Build Path(base path=w1313, name or relative path=w1307) -> (appended path=w1306:path)
                n624 = call "Find_Unique_Filename.vi"("Path In"=w1306) -> ("Unique Path Out"=w1305:path)  [unwired: 1 in, 1 out]
              }
              frame #2 {
                n625 = global read "Extra_Commands_Global.vi" "Minutes Before Repeating Row"() -> (w1318:string)
                n626 = Index Array(array=w1317, index=0) -> (element=w1320:T6)
                n627 = Initialize Array(w1320, 0 ("dimension size")) -> (w1319:T6[])
                n628 = for {
                  shift-right: [w1323] -> w1316
                  shift-left: w1319 -> [w1325]
                  tunnel: w1318 -> [w1327]
                  tunnel: w1317 -> [w1324] mode=indexing
                  n629 = Unbundle By Name(w1324) -> ("Extra Commands"=w1326:string)
                  n630 = call "Extra_Commands.vi"("String to Search"=w1326, "Command"=w1327) -> ("Command Found"=w1328:bool)  [unwired: 1 in, 4 out]
                  n631 = case shown="True" w1328 {
                    tunnel: w1325 -> [w1329 w1332]
                    tunnel: w1324 -> [_ w1331]
                    tunnel: [w1329 w1330] -> w1323
                    frame False {
                    }
                    frame True {
                      n632 = Build Array (concatenate)(w1332, w1331) -> (w1330:T6[])
                    }
                  }
                }
                n633 = Build Array (concatenate)(w1316, w1315) -> (w1314:T6[])
              }
            }
          }
          frame True {
          }
        }
        n634 = Concatenate Strings("Multi run Prog Ended having the setup filename of :" ("Message"), w1280) -> (w1279:string)
        n635 = call "Log_Current_row_to_Execute.vi"("Simulate/Run"=w1278, "Message"=w1279, "Start of Multi Run Prog"=w1275) -> ()  [unwired: 2 in, 5 out]
        n636 = call "Save_Trav_setup.vi"("Work in Tunnel Coordinates?"=w1265, "Trav Table"=w1289, "Jump Bad Positions"=w1264, "Setup filename"=w1291) -> ("Trav Table Out"=w1288:T6[])  [unwired: 1 out]
        n637 = Select(t=w1288, s=w1283, f=w1287) -> (s? t:f=w1286:T6[])
      }
      frame "End" {
        w1337 = ""
        w1339 = path ""
        w1340 = 0 ("No. of pts.")
        w1335 = nan
        n638 = global write "Trav_pos_global.vi" "Estimated Completion time"("") -> ()
        n639 = global write "Trav_pos_global.vi" "Meas Setup Number"(0 ("Meas Setup Number")) -> ()
        n640 = global write "Trav_pos_global.vi" "Top level setup filename"(w1339) -> ()
        n641 = Build Array(u32 0) -> (w1346:u32[])
        n642 = Current VI's Path() -> (path=w1338:path)
        n643 = property on="Table" class="Arr (strict)"("Index Values"=w1346) -> ()  [unwired: 2 in, 2 out]
        n644 = call "Bring_to_front.vi"("path"=w1338) -> ()
        n645 = global read "Trav_pos_global.vi" "Current Row"() -> (w1345:T6)
        n646 = Bundle By Name(cluster=w1345, "Start X"=w1335, "Start Y"=w1335, "Start Z"=w1335, "End X"=w1335, "End Y"=w1335, "End Z"=w1335, "No. of pts."=w1340, "Spacing"=Spacing."Linear", "Filename"=w1339, "Tunnel Speed"=w1335, "Averaging time (min)"=w1335, "Extra Commands"=w1337, "Specific Arguments"=w1337, "Carrier_1 Q (l/min)"=w1335, "Trace Gas Concentration (%)"=w1335, "Carrier_2 Q (l/min)"=w1335, "Comments"=w1337, "Row No"=w1340, "Row Type Selector"=Multi_run_mode."Blank Row", "Completion time"=w1337, "Meas Setup File"=w1337, "Row Duration (mins)"=w1335, "No. of Valid pts."=w1340) -> (w1344:T6)
        n647 = global write "Trav_pos_global.vi" "Current Row"(w1344) -> ()
      }
    }
    n648 = case shown="True" w10 {
      tunnel: w7 -> [_ w17]
      frame False {
      }
      frame True {
        n649 = local write "Table"(w17) -> ()
      }
    }
    "Multi Run Case" <- w12
  }
